vi "HostHoppingScan_v2_MultiRegion.vi"() -> ()   [LabVIEW 2024]
uses:
  <vilib>/Analysis/6fits.llb/Curve Fitting Criteria.ctl
  <vilib>/FPGAPlugInAG/USB-7845R OEM/niLvFpga_Open_USB-7845R OEM.vi
  <vilib>/rvi/interface/common/dynamic/niFpgaDynamicAddResources.vi
  <vilib>/Utility/error.llb/Error Cluster From Error Code.vi
  <vilib>/rvi/errors/niLvFpgaAdjustHostInterfaceError.vi
  <vilib>/rvi/interface/common/niFpgaWaitOnOcc.vi
  <vilib>/FPGAPlugInAG/Dynamic/niLvFpga_Close_Dynamic.vi
  <vilib>/rvi/interface/nirviOpenFPGA/nirviOpenFPGA.xnode
  FPGA Bitfiles/hoppingsicmv2_FPGATarget_FPGAHoppingScanM_mavFg5je4kQ.lvbitx
  <vilib>/rvi/interface/nirviMethod/nirviMethod.xnode
  <vilib>/rvi/interface/nirviReadWriteControl/nirviReadWriteControl.xnode
  <vilib>/rvi/interface/nirviCloseFPGA/nirviCloseFPGA.xnode
  NiFpgaLv.dll
  <vilib>/rvi/interface/Simulation/niFpgaSimulationCallBeginRW.vi
  <vilib>/rvi/errors/niLvFpgaMergeErrorWithErrorCode.vi
  <vilib>/FPGAPlugInAG/Dynamic/niLvFpga_ReadFifo_Dynamic.vi
  <vilib>/FPGAPlugInAG/Dynamic/niLvFpga_WriteFifo_Dynamic.vi
  <vilib>/Analysis/NI_AALPro.lvlib
  <vilib>/FPGAPlugInAG/Dynamic/niLvFpga_ConfigureFifo_Dynamic.vi
panel:
  out "RegionScanning":string
  in  "Auto Image \nSegmentation?":bool
  out "Adapted_YOffset um":dbl format="%#_13g"
  out "Adapted_XOffset um":dbl format="%#_13g"
  out "Adapted_YNum":i32
  out "Adapted_XNum":i32
  in  "Scanning Settings":T1(tab)
  in  "Retract (edge) um":dbl format="%#_13g"
  in  "FrameNum":u32
  in  "XNum":i32
  in  "YNum":i32
  in  "FF_Threshold %":dbl format="%#_13g"
  in  "XStepSize um":dbl format="%#_13g"
  in  "YStepSize um":dbl format="%#_13g"
  in  "YOffset um":dbl format="%#_13g"
  in  "XOffset um":dbl format="%#_13g"
  in  "Retract (flat) um":dbl format="%#_13g"
  in  "RetRate um/s":dbl format="%#_13g"
  in  "FF_AppRate um/s":dbl format="%#_13g"
  in  "NF_AppRate um/s":dbl format="%#_13g"
  in  "Pressure kPa":dbl format="%#_13g"
  in  "NF_Threshold %":dbl format="%#_13g"
  in  "CoordCalThreshold %":dbl format="%#_13g"
  in  "CoordCalRetract um":dbl format="%#_13g"
  in  "YCoordCalEnd um":dbl format="%#_13g"
  in  "XCoordCalEnd um":dbl format="%#_13g"
  in  "YCoordCalBegin um":dbl format="%#_13g"
  in  "XCoordCalBegin um":dbl format="%#_13g"
  in  "CoordCalAppRate um/s":dbl format="%#_13g"
  in  "CoordCalRetRate um/s":dbl format="%#_13g"
  in  "ScanMode":i32(knob) min=0 max=3 scale=0.0..3.0
  out "Signal Size":i32
  out "Done?":bool
  out "HTT_Buffer_Write":u32
  out "Scanned Points":i32
  in  "stop":bool
  in  "Notes":string
  in  "GraphTab":T2(tab)
  out "Topography":dbl[][](graph)
  out "Retract Map":dbl[][](graph)
  out "IZCurve":cluster{dbl[], dbl[]}(graph)
  out "Pressure Slope Map":dbl[][](graph)
  out "FPGA_Host_Buf_Depth":u32
  # "Calibrated Scan\n(New Calibration)"
  # "Calibrated Scan\n(Last Calibration)"
  # "Normal Scan"
  # "Background\nSubstrate Scan"
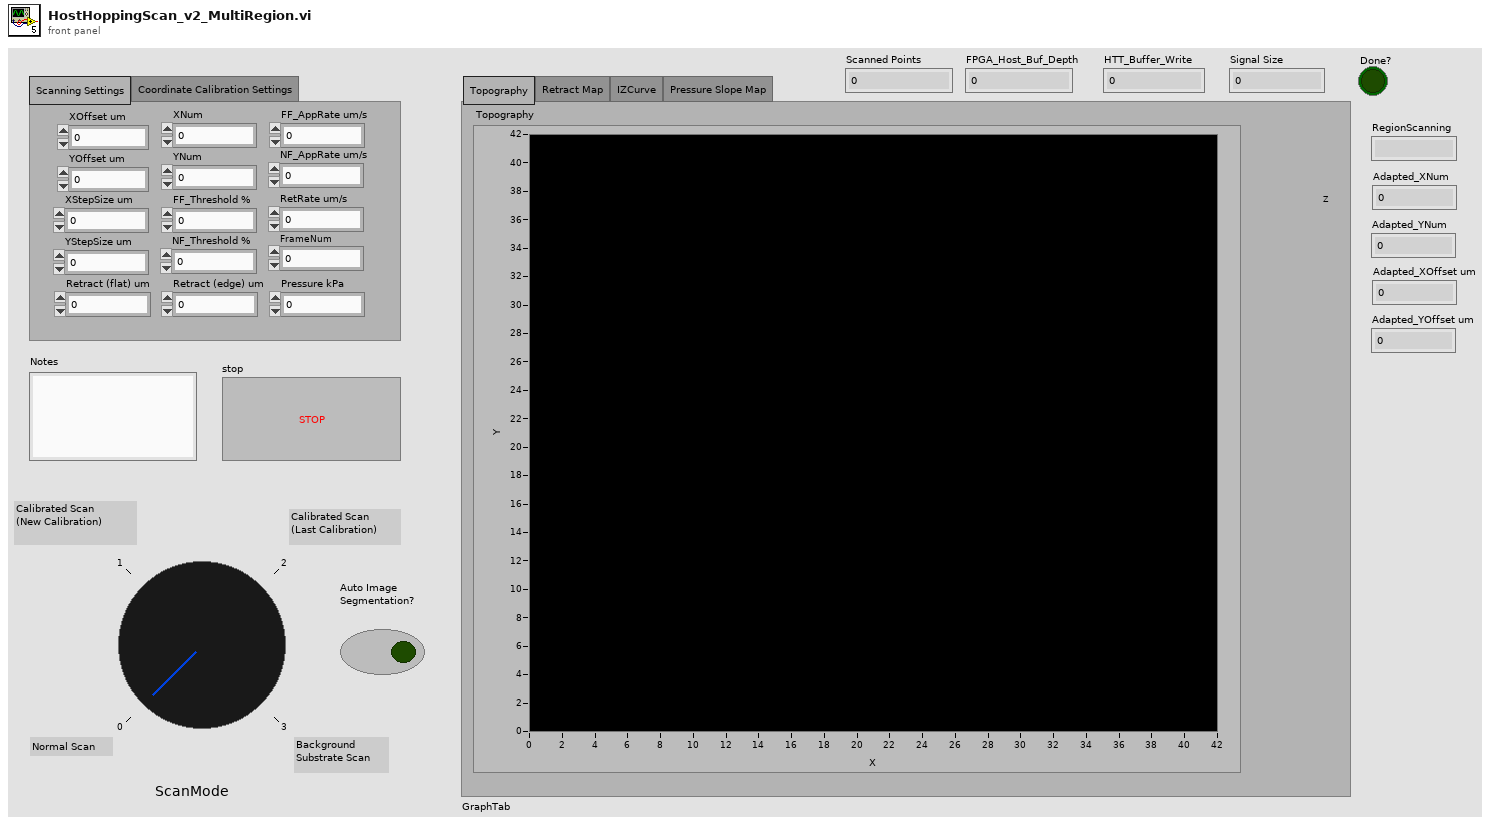
[diagram p1: front panel]
types:
  T1 = enum32{"Scanning Settings", "Coordinate Calibration Settings"}
  T2 = enum32{"Topography", "Retract Map", "IZCurve", "Pressure Slope Map"}
  T3 = typedef "NI_AALPro.lvlib/Curve Fitting Criteria.ctl" = u16
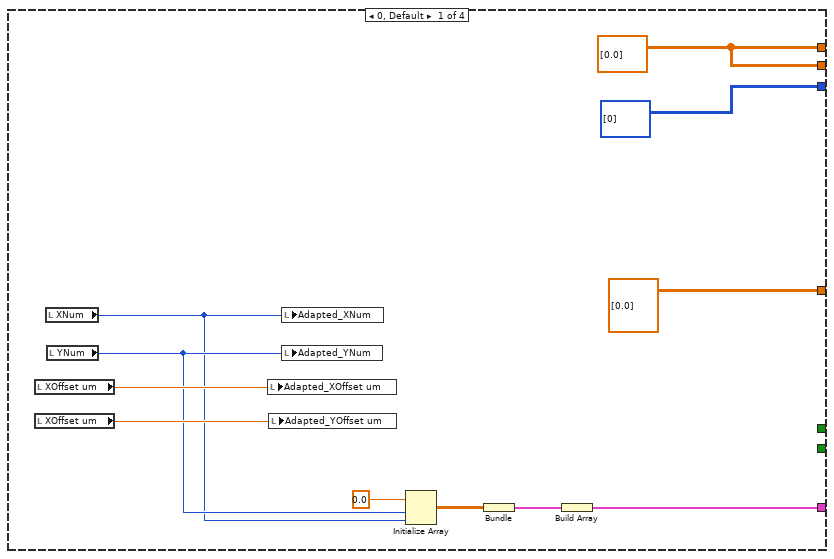
[diagram p3: hidden frame]
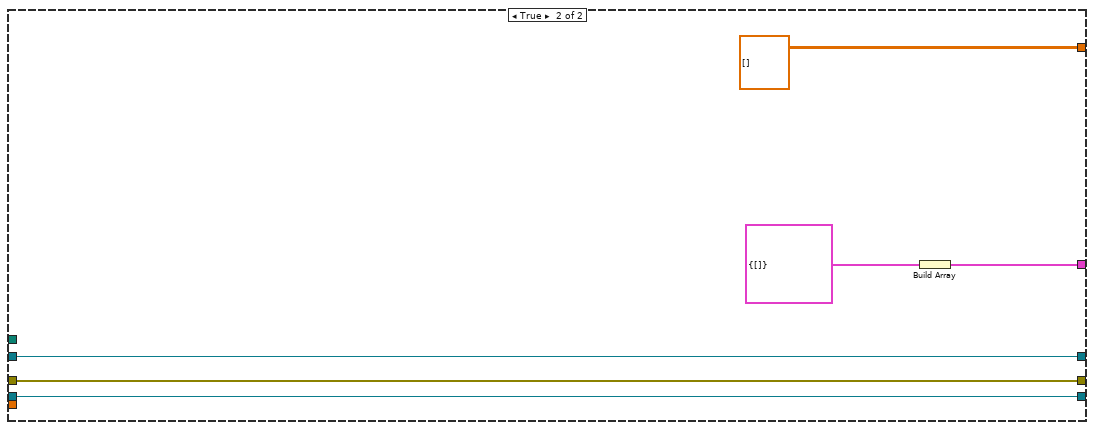
[diagram p4: hidden frame]
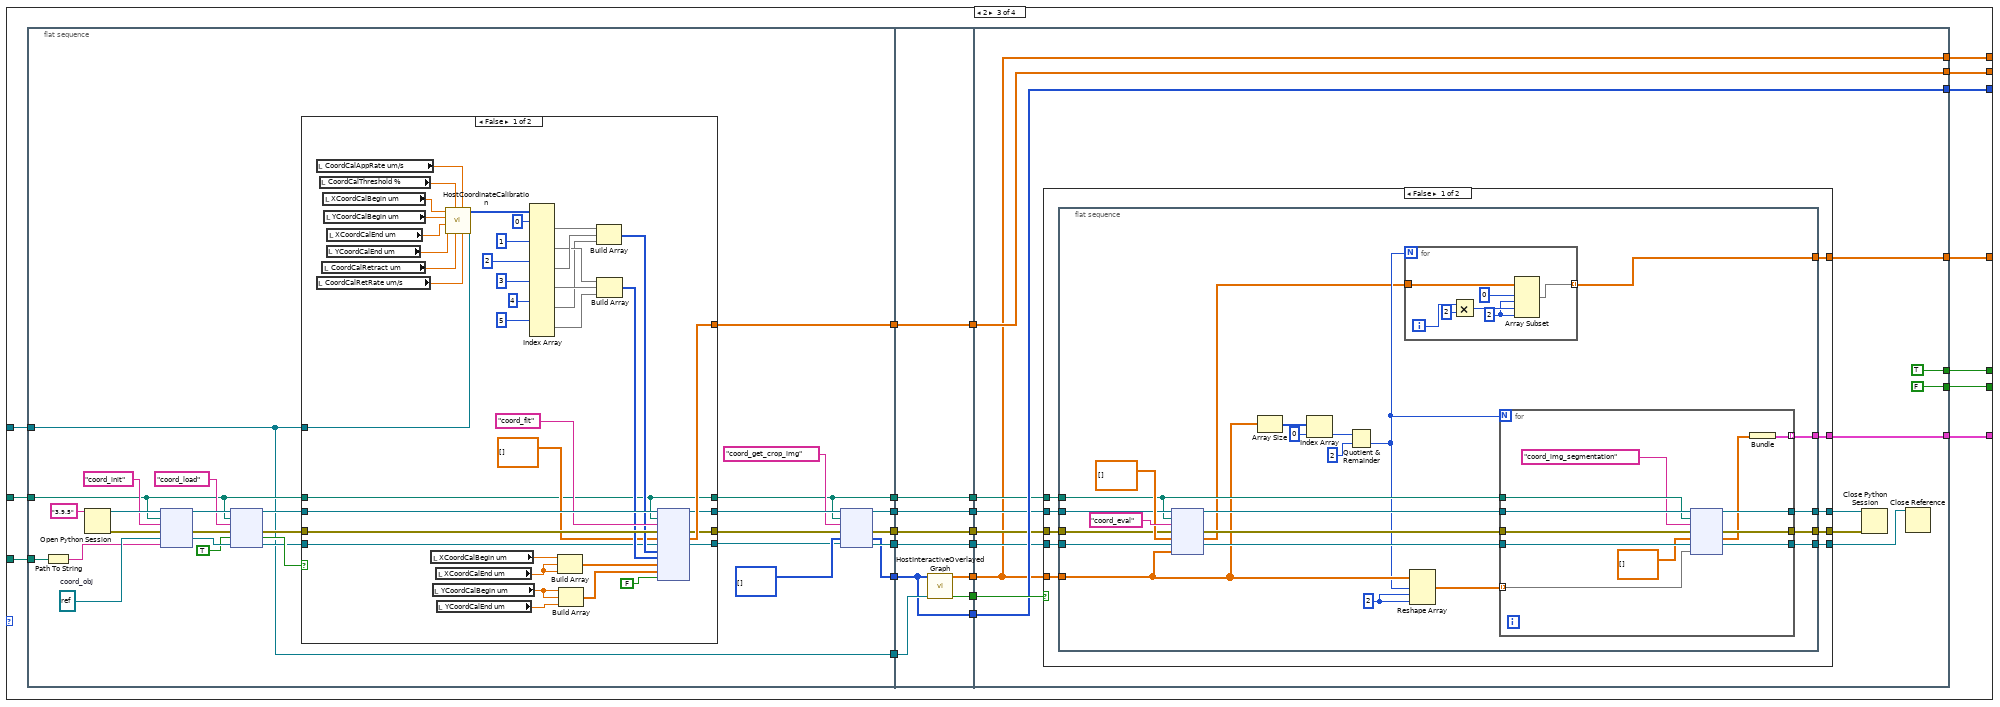
[diagram p5: hidden frame]
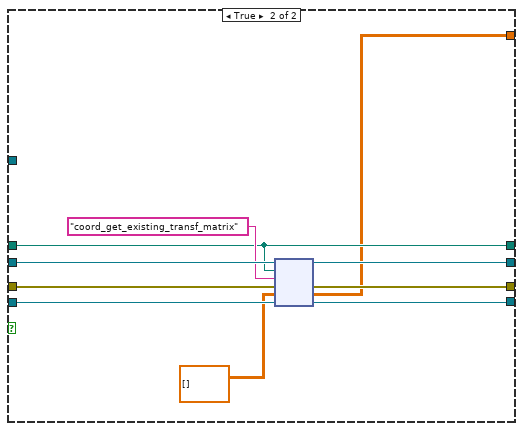
[diagram p6: hidden frame]
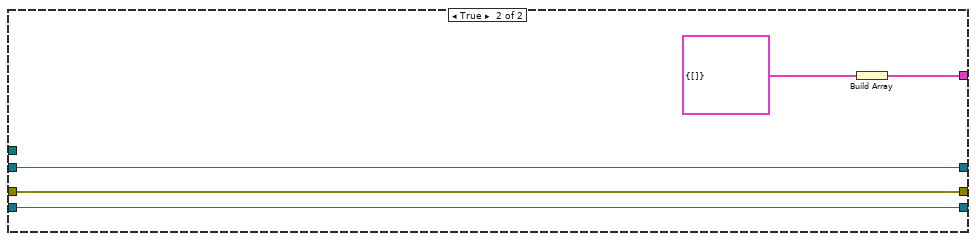
[diagram p7: hidden frame]
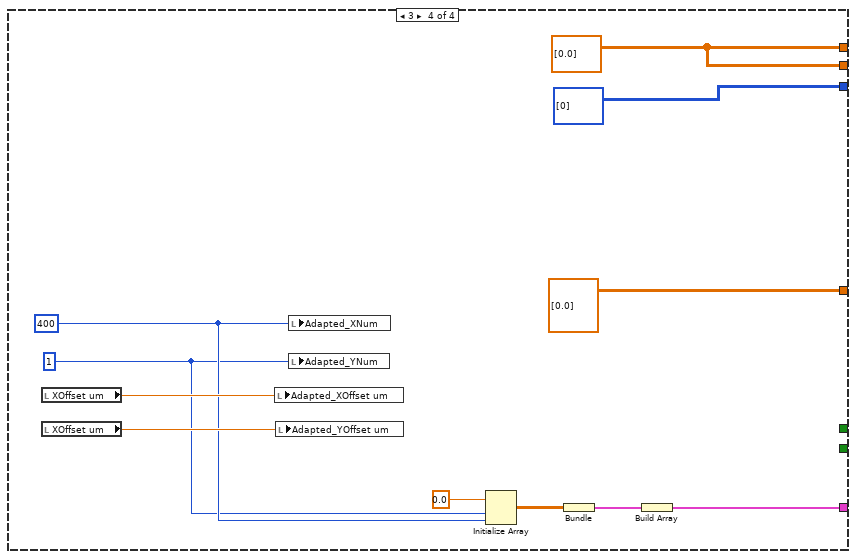
[diagram p8: hidden frame]
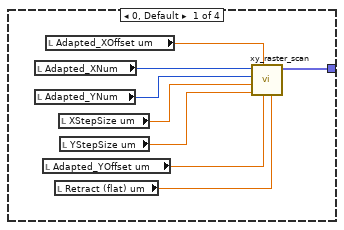
[diagram p14: hidden frame]
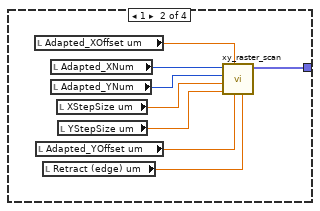
[diagram p15: hidden frame]
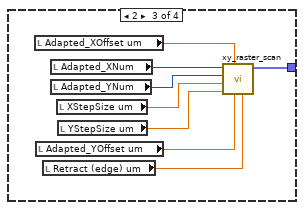
[diagram p16: hidden frame]
diagram:
  n1 = flat-sequence {
    tunnel: [w4] -> w2
    tunnel: w2 -> [w30]
    tunnel: [w27] -> w1
    tunnel: w1 -> [w1436]
    frame #0 {
      n2 = Obtain Queue(max queue size (-1, unlimited)=64, name (unnamed)="stop_sign", element data type=FALSE) -> (queue out=w4:refnum<queue>)  [unwired: 2 in, 2 out]
    }
    frame #1 {
      n3 = flat-sequence {
        tunnel: [w52] -> w31
        tunnel: w30 -> [w52]
        tunnel: w31 -> [w58]
        tunnel: [w58] -> w25
        tunnel: [w54] -> w24
        tunnel: [w107] -> w22
        tunnel: [w108] -> w21
        tunnel: [w109] -> w20
        tunnel: [w110] -> w19
        tunnel: [w111] -> w18
        tunnel: [w74] -> w17
        tunnel: w24 -> [w92]
        tunnel: w25 -> [w74]
        tunnel: [w72] -> w16
        tunnel: [w499] -> w39
        tunnel: [w497] -> w38
        tunnel: [w496] -> w37
        tunnel: [w498] -> w36
        tunnel: [w501] -> w29
        tunnel: w22 -> [w496]
        tunnel: w21 -> [w497]
        tunnel: w20 -> [w499]
        tunnel: w19 -> [w498]
        tunnel: w18 -> [w490]
        tunnel: [w490] -> w23
        tunnel: w17 -> [w494]
        tunnel: w16 -> [w491]
        tunnel: [w491] -> w15
        tunnel: [w489] -> w14
        tunnel: w39 -> [w526]
        tunnel: w38 -> [w525]
        tunnel: w37 -> [w524]
        tunnel: [w522] -> w35
        tunnel: [w521] -> w34
        tunnel: [w520] -> w33
        tunnel: [w519] -> w32
        tunnel: w36 -> [w523]
        tunnel: w29 -> [w518]
        tunnel: [w517] -> w28
        tunnel: w23 -> [w516]
        tunnel: w15 -> [w515]
        tunnel: w14 -> [w514]
        tunnel: [w514] -> w13
        tunnel: [w513] -> w12
        tunnel: [w512] -> w11
        tunnel: [w511] -> w10
        tunnel: [w510] -> w9
        tunnel: [w509] -> w8
        tunnel: [w508] -> w7
        tunnel: w35 -> [w1422]
        tunnel: w34 -> [w1428]
        tunnel: w33 -> [w1427]
        tunnel: w32 -> [w1426]
        tunnel: w28 -> [w1420]
        tunnel: [w1420] -> w26
        tunnel: w13 -> [w1410]
        tunnel: w12 -> [w1409]
        tunnel: w11 -> [w1408]
        tunnel: w10 -> [w1407]
        tunnel: w9 -> [w1406]
        tunnel: w8 -> [w1405]
        tunnel: w7 -> [w1404]
        tunnel: [w1435] -> w27
        tunnel: w26 -> [w1435]
        frame #0 {
          n4 = Wait (ms)(milliseconds to wait=u32 100) -> ()  [unwired: 1 out]
          "Done?" <- FALSE ("Done?")
          "Adapted_XNum" <- "XNum"
          "Adapted_YNum" <- "YNum"
          "Adapted_XOffset um" <- "XStepSize um"
          "Adapted_YOffset um" <- "YStepSize um"
        }
        frame #1 {
          n5 = call "File Dialog"("prompt"="Choose a path to save scanning image data files") -> ("selected path"=w54:path, "cancelled"=w56:bool, "error out"=w55:errorcluster)  [unwired: 11 in, 1 out]
          n6 = Stop(stop? (T)=w56) -> ()
          n7 = call <vilib>:"Clear Errors.vi"("error in (no error)"=w55) -> ()  [unwired: 5 in, 2 out]
        }
        frame #2 {
          w73 = refnum<k38> refnum  # db_obj
          # "coordinate calibration"
          # "use python to save data this time"
          n8 = Path To String(path=w92) -> (string=w106:string)
          n9 = local read "ScanMode"() -> (w75:i32)
          n10 = Get Queue Status(queue=w74) -> (# elements in queue=w91:i32)  [unwired: 2 in, 7 out]
          n11 = Concatenate Strings(w106, "_data.db" ("string")) -> (w105:string)
          n12 = Current VI's Path() -> (path=w97:path)
          n13 = Less Or Equal To 0?(x=w91) -> (x <= 0?=w90:bool)
          n14 = String To Path(string=w105) -> (path=w103:path)
          n15 = Strip Path(path=w97) -> (stripped path=w85:path)  [unwired: 1 out]
          n16 = call <vilib>:"Check if File or Folder Exists.vi"("path"=w103) -> ("file or folder exists?"=w104:bool)  [unwired: 8 in, 2 out]
          n17 = Build Path(base path=w85, name or relative path=path "py/coord_transform.py") -> (appended path=w87:path)
          n18 = Build Path(base path=w85, name or relative path=path "coordinate_calibration/tmp_calibrated_coord") -> (appended path=w84:path)
          n19 = Select(t=w75, s=w90, f=0 ("t")) -> (s? t:f=w89:i32)
          n20 = Build Path(base path=w85, name or relative path=path "py/data_db_arrangement_multi_region.py") -> (appended path=w110:path)
          n21 = case shown="1" w89 {
            tunnel: w87 -> [_ w145 w313 _]
            tunnel: w84 -> [_ w147 w312 _]
            tunnel: w74 -> [_ w146 w311 _]
            tunnel: [w120 w144 w290 w477] -> w111
            tunnel: [i32[][] [[0]] w143 w292 i32[][] [[0]]] -> w60
            tunnel: [w119 w142 w291 w485] -> w61
            tunnel: [w119 w141 w293 w485] -> w62
            tunnel: [_ w140 w294 _] -> w63
            tunnel: [_ w139 w295 _] -> w64
            tunnel: [dbl[][][] [[[0.0]]] ("OutputRetractMap um") w123 w289 dbl[][][] [[[0.0]]] ("OutputRetractMap um")] -> w72
            frame 0, Default {
              w119 = dbl[][] [[0.0]] ("Output_Coord")
              n22 = local read "XOffset um"() -> (w122:dbl)
              n23 = local read "XOffset um"() -> (w121:dbl)
              n24 = local read "XNum"() -> (w112:i32)
              n25 = local read "YNum"() -> (w113:i32)
              n26 = local write "Adapted_XOffset um"(w122) -> ()
              n27 = local write "Adapted_YOffset um"(w121) -> ()
              n28 = local write "Adapted_XNum"(w112) -> ()
              n29 = local write "Adapted_YNum"(w113) -> ()
              n30 = Initialize Array(0.0, w113, w112) -> (w115:dbl[][])
              n31 = Bundle(w115) -> (w114:cluster{dbl[][]})  [unwired: 1 in]
              n32 = Build Array(w114) -> (w120:cluster{dbl[][]}[])
            }
            frame 1 {
              n33 = flat-sequence {
                tunnel: w147 -> [w196]
                tunnel: w146 -> [w149]
                tunnel: w145 -> [w152]
                tunnel: [w152] -> w129
                tunnel: [w160] -> w131
                tunnel: [w155] -> w133
                tunnel: [w154] -> w135
                tunnel: [w153] -> w136
                tunnel: [w150] -> w138
                tunnel: [w149] -> w127
                tunnel: w138 -> [w210]
                tunnel: [w210] -> w137
                tunnel: w136 -> [w202]
                tunnel: w135 -> [w209]
                tunnel: [w209] -> w134
                tunnel: w133 -> [w208]
                tunnel: [w208] -> w132
                tunnel: w131 -> [w207]
                tunnel: [w207] -> w130
                tunnel: w129 -> [w206]
                tunnel: [w206] -> w128
                tunnel: w127 -> [w205]
                tunnel: [w204] -> w126
                tunnel: [w203] -> w125
                tunnel: [w202] -> w124
                tunnel: [w222] -> w144
                tunnel: [w212] -> w143
                tunnel: [w214] -> w142
                tunnel: [w221] -> w141
                tunnel: [TRUE] -> w140
                tunnel: [FALSE] -> w139
                tunnel: w137 -> [w221]
                tunnel: w134 -> [w216]
                tunnel: w132 -> [w217]
                tunnel: w130 -> [w218]
                tunnel: w128 -> [w215]
                tunnel: w126 -> [w214]
                tunnel: w125 -> [w213]
                tunnel: w124 -> [w212]
                tunnel: [w211] -> w123
                frame #0 {
                  w197 = refnum<k38> refnum  # coord_obj
                  # "extended img bundle"
                  # "retracted img bundle"
                  n34 = Path To String(path=w196) -> (string=w195:string)
                  n35 = local read "CoordCalAppRate um/s"() -> (w189:dbl)
                  n36 = local read "CoordCalRetRate um/s"() -> (w187:dbl)
                  n37 = local read "CoordCalThreshold %"() -> (w190:dbl)
                  n38 = local read "CoordCalRetract um"() -> (w188:dbl)
                  n39 = local read "XCoordCalBegin um"() -> (w194:dbl)
                  n40 = local read "YCoordCalBegin um"() -> (w193:dbl)
                  n41 = local read "YCoordCalEnd um"() -> (w191:dbl)
                  n42 = local read "XCoordCalEnd um"() -> (w192:dbl)
                  n43 = Open Python Session(python version="3.9.5" ("Python version")) -> (session out=w200:refnum<k35>, error out=w199:errorcluster)  [unwired: 2 in]
                  n44 = node(w200, w152, "coord_init" ("Python version"), w199, w197, w195) -> (w174:refnum<k35>, w172:errorcluster, w173:refnum<k38>)  [unwired: 1 in, 2 out]
                  n45 = call "HostCoordinateCalibration.vi"("stop_sign_queue"=w149, "RetRate um/s"=w187, "AppRate um/s"=w189, "Retract um"=w188, "Threshold %"=w190, "YCalibrationEnd um"=w191, "XCalibrationEnd um"=w192, "YCalibrationOffset um"=w193, "XCalibrationOffset um"=w194) -> ("img_bundle"=w186:i32[][][])  [unwired: 2 in]
                  n46 = local read "XCoordCalBegin um"() -> (w169:dbl)
                  n47 = local read "YCoordCalBegin um"() -> (w166:dbl)
                  n48 = local read "XCoordCalEnd um"() -> (w168:dbl)
                  n49 = local read "YCoordCalEnd um"() -> (w167:dbl)
                  n50 = Index Array(array=w186, index (dim 0) #1=0 ("index (page)"), index (dim 0) #2=1 ("index (page)"), index (dim 0) #3=2 ("index (page)"), index (dim 0) #4=3 ("index (page)"), index (dim 0) #5=4 ("index (page)"), index (dim 0) #6=5 ("index (page)")) -> (element #1=w148:i32[][], element #2=w178:i32[][], element #3=w179:i32[][], element #4=w177:i32[][], element #5=w176:i32[][], element #6=w175:i32[][])  [unwired: 12 in]
                  n51 = Build Array(w169, w168, w168) -> (w165:dbl[])
                  n52 = Build Array(w166, w166, w167) -> (w164:dbl[])
                  n53 = Build Array(w148, w179, w176) -> (w171:i32[][][])
                  n54 = Build Array(w178, w177, w175) -> (w170:i32[][][])
                  n55 = node(w174, w152, "coord_fit" ("function name"), w172, dbl[][] [], w173, w171, w170, w165, w164, TRUE) -> (w161:refnum<k35>, w159:errorcluster, w150:dbl[][], w157:refnum<k38>)  [unwired: 5 in, 2 out]
                  n56 = node(w161, w152, "coord_get_crop_img" ("function name"), w159, i32[][] [], w157) -> (w160:refnum<k35>, w155:errorcluster, w153:i32[][], w154:refnum<k38>)  [unwired: 2 out]
                }
                frame #1 {
                  n57 = call "HostInteractiveOverlayedGraph.vi"("stop_sign_queue"=w205, "InputImg"=w202) -> ("Break"=w203:bool, "Output_Coord"=w204:dbl[][])  [unwired: 8 in]
                }
                frame #2 {
                  n58 = case shown="False" w213 {
                    tunnel: [w235 w288] -> w225
                    tunnel: [w234 w287] -> w224
                    tunnel: [w233 w286] -> w223
                    tunnel: [w227 w283] -> w222
                    tunnel: w214 -> [w232 _]
                    tunnel: w218 -> [w231 w288]
                    tunnel: w217 -> [w230 w287]
                    tunnel: w216 -> [w229 w286]
                    tunnel: w215 -> [w228 _]
                    tunnel: [w226 dbl[][][] [] ("OutputRetractMap um")] -> w211
                    frame False {
                      n59 = flat-sequence {
                        tunnel: [w245] -> w227
                        tunnel: [w255] -> w233
                        tunnel: [w256] -> w234
                        tunnel: [w257] -> w235
                        tunnel: w228 -> [w246]
                        tunnel: w229 -> [w252]
                        tunnel: w230 -> [w253]
                        tunnel: w231 -> [w254]
                        tunnel: w232 -> [w237]
                        tunnel: [w239] -> w226
                        frame #0 {
                          n60 = node(w254, w246, "coord_eval" ("function name"), w253, dbl[][] [], w252, w237) -> (w249:refnum<k35>, w248:errorcluster, w240:dbl[][], w247:refnum<k38>)  [unwired: 1 in, 2 out]
                          n61 = Array Size(array=w237) -> (size(s)=w244:i32[])
                          n62 = Index Array(array=w244, index=0) -> (element=w242:i32)
                          n63 = Quotient & Remainder(x=w242, y=2 ("index")) -> (floor(x/y)=w238:i32)  [unwired: 1 out]
                          n64 = for {
                            N: w238 -> [_]
                            tunnel: w237 -> [w263]
                            tunnel: [w258] -> w236 mode=indexing
                            i -> [w262]
                            n65 = Multiply(x=w262, y=2) -> (x*y=w260:i32)
                            n66 = Array Subset(array=w263, index (row)=w260, length (row)=2 ("length")) -> (w258:dbl[][])  [unwired: 2 in]
                          }
                          n67 = for {
                            N: w238 -> [_]
                            tunnel: w240 -> [w267]
                            tunnel: [w266] -> w239 mode=indexing
                            i -> [w264]
                            w268 = 2 ("length")
                            n68 = Multiply(x=2 ("y"), y=w264) -> (x*y=w270:i32)
                            n69 = Array Subset(array=w267, index (row)=0 ("index"), length (row)=w268, index (col)=w270, length (col)=w268) -> (w266:dbl[][])
                          }
                          n70 = for {
                            N: w238 -> [_]
                            tunnel: w236 -> [w279] mode=indexing
                            tunnel: w246 -> [w273]
                            tunnel: [w271] -> w245 mode=indexing
                            tunnel: w249 -> [w278]
                            tunnel: [w282] -> w257
                            tunnel: w248 -> [w277]
                            tunnel: [w281] -> w256
                            tunnel: w247 -> [w276]
                            tunnel: [w280] -> w255
                            n71 = node(w278, w273, "coord_img_segmentation" ("function name"), w277, dbl[][] [], w276, w279) -> (w282:refnum<k35>, w281:errorcluster, w272:dbl[][], w280:refnum<k38>)  [unwired: 1 in, 2 out]
                            n72 = Bundle(w272) -> (w271:cluster{dbl[][]})  [unwired: 1 in]
                          }
                        }
                      }
                    }
                    frame True {
                      n73 = Build Array(cluster{dbl[][]} {[]}) -> (w283:cluster{dbl[][]}[])
                    }
                  }
                  n74 = Close Python Session(session in=w225, error in=w224) -> ()  [unwired: 1 out]
                  n75 = Close Reference(reference=w223) -> ()  [unwired: 1 in, 1 out]
                }
              }
            }
            frame 2 {
              n76 = flat-sequence {
                tunnel: w313 -> [w327]
                tunnel: w312 -> [w336]
                tunnel: w311 -> [w325]
                tunnel: [w314] -> w310
                tunnel: [w325] -> w309
                tunnel: [w324] -> w308
                tunnel: [w318] -> w305
                tunnel: [w317] -> w303
                tunnel: [w316] -> w301
                tunnel: [w315] -> w299
                tunnel: w310 -> [w394]
                tunnel: w309 -> [w402]
                tunnel: w308 -> [w401]
                tunnel: [w401] -> w307
                tunnel: [w400] -> w306
                tunnel: w305 -> [w400]
                tunnel: [w399] -> w304
                tunnel: w303 -> [w399]
                tunnel: [w398] -> w302
                tunnel: w301 -> [w398]
                tunnel: [w397] -> w300
                tunnel: w299 -> [w397]
                tunnel: [w396] -> w298
                tunnel: [w395] -> w297
                tunnel: [w394] -> w296
                tunnel: w307 -> [w414]
                tunnel: w306 -> [w412]
                tunnel: w304 -> [w411]
                tunnel: w302 -> [w410]
                tunnel: w300 -> [w409]
                tunnel: w298 -> [w408]
                tunnel: w297 -> [w417]
                tunnel: w296 -> [w413]
                tunnel: [FALSE] -> w295
                tunnel: [TRUE] -> w294
                tunnel: [w414] -> w293
                tunnel: [w413] -> w292
                tunnel: [w408] -> w291
                tunnel: [w404] -> w290
                tunnel: [w403] -> w289
                frame #0 {
                  w338 = refnum<k38> refnum  # coord_obj
                  n77 = Path To String(path=w336) -> (string=w337:string)
                  n78 = Open Python Session(python version="3.9.5" ("Python version")) -> (session out=w341:refnum<k35>, error out=w340:errorcluster)  [unwired: 2 in]
                  n79 = node(w341, w327, "coord_init" ("Python version"), w340, w338, w337) -> (w335:refnum<k35>, w334:errorcluster, w333:refnum<k38>)  [unwired: 1 in, 2 out]
                  n80 = node(w335, w327, "coord_load" ("Python version"), w334, TRUE, w333) -> (w329:refnum<k35>, w328:errorcluster, w330:bool, w326:refnum<k38>)  [unwired: 2 out]
                  n81 = case shown="False" w330 {
                    tunnel: w329 -> [w361 w393]
                    tunnel: w328 -> [w359 w392]
                    tunnel: w325 -> [w375 _]
                    tunnel: w327 -> [w343 w385]
                    tunnel: w326 -> [w349 w391]
                    tunnel: [w347 w384] -> w324
                    tunnel: [w346 w388] -> w323
                    tunnel: [w345 w387] -> w320
                    tunnel: [w344 w386] -> w319
                    tunnel: [w343 w385] -> w318
                    frame False {
                      n82 = local read "CoordCalAppRate um/s"() -> (w378:dbl)
                      n83 = local read "CoordCalRetRate um/s"() -> (w376:dbl)
                      n84 = local read "CoordCalThreshold %"() -> (w379:dbl)
                      n85 = local read "CoordCalRetract um"() -> (w377:dbl)
                      n86 = local read "XCoordCalBegin um"() -> (w383:dbl)
                      n87 = local read "YCoordCalBegin um"() -> (w382:dbl)
                      n88 = local read "YCoordCalEnd um"() -> (w380:dbl)
                      n89 = local read "XCoordCalEnd um"() -> (w381:dbl)
                      n90 = local read "XCoordCalBegin um"() -> (w358:dbl)
                      n91 = local read "YCoordCalBegin um"() -> (w355:dbl)
                      n92 = local read "XCoordCalEnd um"() -> (w357:dbl)
                      n93 = local read "YCoordCalEnd um"() -> (w356:dbl)
                      n94 = call "HostCoordinateCalibration.vi"("stop_sign_queue"=w375, "RetRate um/s"=w376, "AppRate um/s"=w378, "Retract um"=w377, "Threshold %"=w379, "YCalibrationEnd um"=w380, "XCalibrationEnd um"=w381, "YCalibrationOffset um"=w382, "XCalibrationOffset um"=w383) -> ("img_bundle"=w362:i32[][][])  [unwired: 2 in]
                      n95 = Index Array(array=w362, index (dim 0) #1=0 ("index (page)"), index (dim 0) #2=1 ("index (page)"), index (dim 0) #3=2 ("index (page)"), index (dim 0) #4=3 ("index (page)"), index (dim 0) #5=4 ("index (page)"), index (dim 0) #6=5 ("index (page)")) -> (element #1=w363:i32[][], element #2=w367:i32[][], element #3=w368:i32[][], element #4=w366:i32[][], element #5=w365:i32[][], element #6=w364:i32[][])  [unwired: 12 in]
                      n96 = Build Array(w358, w357, w357) -> (w352:dbl[])
                      n97 = Build Array(w355, w355, w356) -> (w351:dbl[])
                      n98 = Build Array(w363, w368, w365) -> (w354:i32[][][])
                      n99 = Build Array(w367, w366, w364) -> (w353:i32[][][])
                      n100 = node(w361, w343, "coord_fit" ("function name"), w359, dbl[][] [], w349, w354, w353, w352, w351, FALSE) -> (w346:refnum<k35>, w345:errorcluster, w347:dbl[][], w344:refnum<k38>)  [unwired: 5 in, 2 out]
                    }
                    frame True {
                      n101 = node(w393, w385, "coord_get_existing_transf_matrix" ("Python version"), w392, dbl[][] [], w391) -> (w388:refnum<k35>, w387:errorcluster, w384:dbl[][], w386:refnum<k38>)  [unwired: 2 out]
                    }
                  }
                  n102 = node(w323, w318, "coord_get_crop_img" ("function name"), w320, i32[][] [], w319) -> (w317:refnum<k35>, w316:errorcluster, w314:i32[][], w315:refnum<k38>)  [unwired: 2 out]
                }
                frame #1 {
                  n103 = call "HostInteractiveOverlayedGraph.vi"("stop_sign_queue"=w402, "InputImg"=w394) -> ("Break"=w395:bool, "Output_Coord"=w396:dbl[][])  [unwired: 8 in]
                }
                frame #2 {
                  n104 = case shown="False" w417 {
                    tunnel: w412 -> [w427 _]
                    tunnel: w411 -> [w426 w474]
                    tunnel: w410 -> [w425 w473]
                    tunnel: w409 -> [w424 w472]
                    tunnel: w408 -> [w423 _]
                    tunnel: [w422 w474] -> w407
                    tunnel: [w421 w473] -> w406
                    tunnel: [w420 w472] -> w405
                    tunnel: [w419 w470] -> w404
                    tunnel: [w418 _] -> w403
                    frame False {
                      n105 = flat-sequence {
                        tunnel: [w450] -> w422
                        tunnel: [w449] -> w421
                        tunnel: [w448] -> w420
                        tunnel: [w447] -> w419
                        tunnel: w423 -> [w432]
                        tunnel: w424 -> [w442]
                        tunnel: w425 -> [w443]
                        tunnel: w426 -> [w444]
                        tunnel: w427 -> [w438]
                        tunnel: [w429] -> w418
                        frame #0 {
                          w433 = 2 ("index")
                          n106 = node(w444, w438, "coord_eval" ("function name"), w443, dbl[][] [], w442, w432) -> (w441:refnum<k35>, w440:errorcluster, w428:dbl[][], w439:refnum<k38>)  [unwired: 1 in, 2 out]
                          n107 = Array Size(array=w432) -> (size(s)=w437:i32[])
                          n108 = Index Array(array=w437, index=0) -> (element=w435:i32)
                          n109 = Quotient & Remainder(x=w435, y=2 ("index")) -> (floor(x/y)=w430:i32)  [unwired: 1 out]
                          n110 = for {
                            N: w430 -> [_]
                            tunnel: w428 -> [w457]
                            tunnel: [w454] -> w429 mode=indexing
                            i -> [w456]
                            w451 = 2 ("length")
                            n111 = Multiply(x=w456, y=2) -> (x*y=w453:i32)
                            n112 = Array Subset(array=w457, index (row)=0 ("index"), length (row)=w451, index (col)=w453, length (col)=w451) -> (w454:dbl[][])
                          }
                          n113 = Reshape Array(w432, w430, w433, w433) -> (w431:dbl[][][])
                          n114 = for {
                            N: w430 -> [_]
                            tunnel: w431 -> [w466] mode=indexing
                            tunnel: w438 -> [w465]
                            tunnel: [w458] -> w447 mode=indexing
                            tunnel: w441 -> [w469]
                            tunnel: [w464] -> w450
                            tunnel: w440 -> [w468]
                            tunnel: [w462] -> w449
                            tunnel: w439 -> [w467]
                            tunnel: [w461] -> w448
                            n115 = node(w469, w465, "coord_img_segmentation" ("function name"), w468, dbl[][] [], w467, w466) -> (w464:refnum<k35>, w462:errorcluster, w459:dbl[][], w461:refnum<k38>)  [unwired: 1 in, 2 out]
                            n116 = Bundle(w459) -> (w458:cluster{dbl[][]})  [unwired: 1 in]
                          }
                        }
                      }
                    }
                    frame True {
                      n117 = Build Array(cluster{dbl[][]} {[]}) -> (w470:cluster{dbl[][]}[])
                    }
                  }
                  n118 = Close Python Session(session in=w407, error in=w406) -> ()  [unwired: 1 out]
                  n119 = Close Reference(reference=w405) -> ()  [unwired: 1 in, 1 out]
                }
              }
            }
            frame 3 {
              w475 = 1 ("Adapted_XNum")
              w476 = 400 ("Adapted_XNum")
              w485 = dbl[][] [[0.0]] ("Output_Coord")
              n120 = local read "XOffset um"() -> (w482:dbl)
              n121 = local read "XOffset um"() -> (w481:dbl)
              n122 = local write "Adapted_XOffset um"(w482) -> ()
              n123 = local write "Adapted_YOffset um"(w481) -> ()
              n124 = local write "Adapted_XNum"(w476) -> ()
              n125 = local write "Adapted_YNum"(w475) -> ()
              n126 = Initialize Array(0.0, w475, w476) -> (w479:dbl[][])
              n127 = Bundle(w479) -> (w478:cluster{dbl[][]})  [unwired: 1 in]
              n128 = Build Array(w478) -> (w477:cluster{dbl[][]}[])
            }
          }
          n129 = case shown="True" w104 {
            tunnel: w103 -> [w486 w488]
            tunnel: [w486 w487] -> w102
            frame False {
            }
            frame True {
              n130 = Delete(path (use dialog)=w488) -> (deleted path=w487:path)  [unwired: 4 in, 2 out]
            }
          }
          n131 = Path To String(path=w102) -> (string=w94:string)
          n132 = Open Python Session(python version="3.9.5" ("Python version")) -> (session out=w99:refnum<k35>, error out=w98:errorcluster)  [unwired: 2 in]
          n133 = node(w99, w110, "db_init" ("Python version"), w98, w73, w94) -> (w83:refnum<k35>, w82:errorcluster, w81:refnum<k38>)  [unwired: 1 in, 2 out]
          n134 = local read "CoordCalAppRate um/s"() -> (w65:dbl)
          n135 = local read "CoordCalRetRate um/s"() -> (w59:dbl)
          n136 = local read "CoordCalThreshold %"() -> (w67:dbl)
          n137 = local read "CoordCalRetract um"() -> (w66:dbl)
          n138 = local read "XCoordCalBegin um"() -> (w71:dbl)
          n139 = local read "YCoordCalBegin um"() -> (w70:dbl)
          n140 = local read "YCoordCalEnd um"() -> (w68:dbl)
          n141 = local read "XCoordCalEnd um"() -> (w69:dbl)
          n142 = node(w83, w110, "db_insert_coordinate_calibration" ("function name"), w82, w81, w71, w70, w69, w68, w67, w66, w65, w59, w60, w61, w62, w63, w64) -> (w80:refnum<k35>, w79:errorcluster, w78:refnum<k38>)  [unwired: 15 in, 2 out]
          n143 = node(w80, w110, "db_start_global_timer" ("function name"), w79, w78) -> (w109:refnum<k35>, w108:errorcluster, w107:refnum<k38>)  [unwired: 2 in, 2 out]
        }
        frame #3 {
          n144 = Get Queue Status(queue=w494) -> (queue out=w493:refnum<queue>, # elements in queue=w495:i32)  [unwired: 2 in, 6 out]
          n145 = Greater Than 0?(x=w495) -> (x > 0?=w492:bool)
          n146 = case shown="True" w492 {
            tunnel: w493 -> [w502 w505]
            tunnel: [w502 w503] -> w501
            frame False {
            }
            frame True {
              n147 = flat-sequence {
                tunnel: w505 -> [w506]
                tunnel: [w506] -> w504
                tunnel: w504 -> [w507]
                tunnel: [w507] -> w503
                frame #0 {
                  n148 = Release Queue(queue=w506) -> ()  [unwired: 2 in, 3 out]
                }
                frame #1 {
                  n149 = Stop() -> ()  [unwired: 1 in]
                }
              }
            }
          }
          n150 = Array Size(array=w490) -> (size(s)=w489:i32)
          n151 = Wait (ms)(milliseconds to wait=u32 200) -> ()  [unwired: 1 out]
        }
        frame #4 {
          n152 = for {
            N: w514 -> [_]
            tunnel: w516 -> [w559] mode=indexing
            tunnel: w523 -> [w566]
            tunnel: [w565] -> w522
            tunnel: w526 -> [w569]
            tunnel: [w564] -> w521
            tunnel: w525 -> [w568]
            tunnel: [w563] -> w520
            tunnel: w524 -> [w567]
            tunnel: [w562] -> w519
            tunnel: w518 -> [w561]
            tunnel: [w560] -> w517
            tunnel: w515 -> [w545] mode=indexing
            tunnel: w514 -> [w541]
            tunnel: [w532] -> w513 mode=indexing
            tunnel: [w531] -> w512 mode=indexing
            tunnel: [w530] -> w511 mode=indexing
            tunnel: [w529] -> w510 mode=indexing
            tunnel: [w528] -> w509 mode=indexing
            tunnel: [w527] -> w508 mode=indexing
            i -> [w544]
            stop <- w546 stop-if-true
            n153 = flat-sequence {
              tunnel: w559 -> [w577]
              tunnel: w561 -> [w586]
              tunnel: w566 -> [w587]
              tunnel: w567 -> [w588]
              tunnel: w568 -> [w589]
              tunnel: w569 -> [w590]
              tunnel: [w590] -> w558
              tunnel: [w589] -> w556
              tunnel: [w588] -> w554
              tunnel: [w587] -> w552
              tunnel: [w586] -> w550
              tunnel: [w576] -> w548
              tunnel: w545 -> [w585]
              tunnel: w544 -> [w582]
              tunnel: [w582] -> w542
              tunnel: w541 -> [w584]
              tunnel: [w584] -> w539
              tunnel: w558 -> [w638]
              tunnel: [w638] -> w557
              tunnel: w556 -> [w637]
              tunnel: [w637] -> w555
              tunnel: w554 -> [w636]
              tunnel: [w636] -> w553
              tunnel: w552 -> [w635]
              tunnel: [w635] -> w551
              tunnel: w550 -> [w634]
              tunnel: [w634] -> w549
              tunnel: w548 -> [w629]
              tunnel: [w628] -> w547
              tunnel: [w627] -> w543
              tunnel: w542 -> [w627]
              tunnel: [w626] -> w540
              tunnel: w539 -> [w626]
              tunnel: w557 -> [w652]
              tunnel: w555 -> [w651]
              tunnel: w553 -> [w650]
              tunnel: w551 -> [w649]
              tunnel: w549 -> [w644]
              tunnel: w547 -> [w642]
              tunnel: w543 -> [w640]
              tunnel: w540 -> [w639]
              tunnel: [w648] -> w538
              tunnel: [w647] -> w537
              tunnel: [w646] -> w536
              tunnel: [w645] -> w535
              tunnel: [w643] -> w534
              tunnel: [w641] -> w533
              tunnel: [w1398] -> w546
              tunnel: [w1399] -> w560
              tunnel: [w1400] -> w562
              tunnel: [w1401] -> w563
              tunnel: [w1402] -> w564
              tunnel: [w1403] -> w565
              tunnel: w538 -> [w1403]
              tunnel: w537 -> [w1402]
              tunnel: w536 -> [w1401]
              tunnel: w535 -> [w1400]
              tunnel: w534 -> [w1399]
              tunnel: w533 -> [w1398]
              tunnel: [w1397] -> w532
              tunnel: [w1396] -> w531
              tunnel: [w1395] -> w530
              tunnel: [w1394] -> w529
              tunnel: [w1393] -> w528
              tunnel: [w1392] -> w527
              frame #0 {
                n154 = local read "ScanMode"() -> (w573:i32)
                n155 = Equal?(x=w573, y=1) -> (x = y?=w572:bool)
                n156 = Equal?(x=w573, y=2) -> (x = y?=w571:bool)
                n157 = Unbundle(w577) -> (w576:dbl[][])
                n158 = Or(x=w572, y=w571) -> (x .or. y?=w570:bool)
                n159 = case shown="True" w570 {
                  tunnel: w585 -> [_ w599]
                  frame False {
                  }
                  frame True {
                    n160 = local read "YCoordCalBegin um"() -> (w617:dbl)
                    n161 = Index Array(array=w599, index (col) #1=0 ("index (row)"), index (col) #2=1 ("index (row)")) -> (element #1=w625:dbl[], element #2=w624:dbl[])  [unwired: 2 in]
                    n162 = local read "YCoordCalEnd um"() -> (w618:dbl)
                    n163 = Index Array(array=w625, index #1=0 ("index"), index #2=1 ("index")) -> (element #1=w623:dbl, element #2=w621:dbl)
                    n164 = Index Array(array=w624, index #1=0 ("index"), index #2=1 ("index")) -> (element #1=w622:dbl, element #2=w620:dbl)
                    n165 = local read "YStepSize um"() -> (w606:dbl)
                    n166 = local read "XStepSize um"() -> (w612:dbl)
                    n167 = Max & Min(x=w623, y=w622) -> (max(x,y)=w614:dbl, min(x,y)=w596:dbl)
                    n168 = Max & Min(x=w621, y=w620) -> (max(x,y)=w597:dbl, min(x,y)=w598:dbl)
                    n169 = Subtract(x=w618, y=w617) -> (x-y=w619:dbl)
                    n170 = Subtract(x=w614, y=w596) -> (x-y=w613:dbl)
                    n171 = Subtract(x=w619, y=w597) -> (x-y=w592:dbl)
                    n172 = Subtract(x=w597, y=w598) -> (x-y=w607:dbl)
                    n173 = Divide(x=w613, y=w612) -> (x/y=w616:dbl)
                    n174 = Divide(x=w607, y=w606) -> (x/y=w608:dbl)
                    n175 = Subtract(x=w596, y=1.0) -> (x-y=w595:dbl)
                    n176 = Subtract(x=w592, y=0.0) -> (x-y=w591:dbl)
                    n177 = Round To Nearest(number=w616) -> (nearest integer value=w615:dbl)
                    n178 = Round To Nearest(number=w608) -> (nearest integer value=w609:dbl)
                    n179 = local write "Adapted_XOffset um"(w595) -> ()
                    n180 = To Long Integer(number=w615) -> (32bit integer=w611:i32)
                    n181 = To Long Integer(number=w609) -> (32bit integer=w610:i32)
                    n182 = local write "Adapted_YOffset um"(w591) -> ()
                    n183 = local write "Adapted_XNum"(w611) -> ()
                    n184 = local write "Adapted_YNum"(w610) -> ()
                  }
                }
                n185 = Increment(x=w582) -> (x+1=w581:i32)
                n186 = Number To Decimal String(number=w584) -> (decimal integer string=w580:string)  [unwired: 1 in]
                n187 = Number To Decimal String(number=w581) -> (decimal integer string=w579:string)  [unwired: 1 in]
                n188 = Concatenate Strings(w579, " / " ("string"), w580) -> (w583:string)
                n189 = local write "RegionScanning"(w583) -> ()
              }
              frame #1 {
                n190 = local read "Adapted_XNum"() -> (w633:i32)
                n191 = local read "Adapted_YNum"() -> (w632:i32)
                n192 = local read "Retract (edge) um"() -> (w630:dbl)
                n193 = local read "Retract (flat) um"() -> (w631:dbl)
                n194 = call "HostDynamicRetractFormalization.vi"("Retract_Edge um"=w630, "Retract_Flat um"=w631, "YNum"=w632, "XNum"=w633, "InputLabel"=w629) -> ("OutputRetractMap um"=w628:dbl[][])  [unwired: 6 in]
                n195 = local write "Retract Map"(w628) -> ()
              }
              frame #2 {
                n196 = local read "FrameNum"() -> (w653:u32)
                n197 = for {
                  N: w653 -> [_]
                  tunnel: w652 -> [w687]
                  tunnel: w651 -> [w686]
                  tunnel: w650 -> [w685]
                  tunnel: w649 -> [w684]
                  tunnel: [w673] -> w648
                  tunnel: [w672] -> w647
                  tunnel: [w671] -> w646
                  tunnel: [w670] -> w645
                  tunnel: w644 -> [w667]
                  tunnel: [w664] -> w643
                  tunnel: w642 -> [w661]
                  tunnel: [w659] -> w641
                  tunnel: w640 -> [w658]
                  tunnel: w639 -> [w656]
                  i -> [w683]
                  stop <- w659 stop-if-true
                  n198 = flat-sequence {
                    tunnel: w683 -> [w706]
                    tunnel: w684 -> [w699]
                    tunnel: w685 -> [w701]
                    tunnel: w686 -> [w702]
                    tunnel: w687 -> [w703]
                    tunnel: [w700] -> w682
                    tunnel: [w698] -> w681
                    tunnel: [w697] -> w680
                    tunnel: [w699] -> w679
                    tunnel: [w706] -> w678
                    tunnel: w667 -> [w695]
                    tunnel: [w695] -> w666
                    tunnel: w661 -> [w693]
                    tunnel: [w693] -> w660
                    tunnel: w658 -> [w690]
                    tunnel: [w690] -> w657
                    tunnel: w656 -> [w689]
                    tunnel: [w689] -> w655
                    tunnel: [w752] -> w688
                    tunnel: w682 -> [w747]
                    tunnel: w681 -> [w746]
                    tunnel: w680 -> [w745]
                    tunnel: w679 -> [w744]
                    tunnel: w678 -> [w712]
                    tunnel: [w739] -> w677
                    tunnel: [w738] -> w676
                    tunnel: [w737] -> w675
                    tunnel: [w736] -> w674
                    tunnel: [w735] -> w669
                    tunnel: [w734] -> w668
                    tunnel: w666 -> [w724]
                    tunnel: [w723] -> w665
                    tunnel: [w719] -> w663
                    tunnel: [w718] -> w662
                    tunnel: w660 -> [w713]
                    tunnel: w657 -> [w711]
                    tunnel: w655 -> [w710]
                    tunnel: [w707] -> w654
                    tunnel: w688 -> [w1391]
                    tunnel: w677 -> [w1386]
                    tunnel: w676 -> [w1388]
                    tunnel: w675 -> [w1387]
                    tunnel: w674 -> [w1383]
                    tunnel: [w1386] -> w673
                    tunnel: [w1385] -> w672
                    tunnel: [w1384] -> w671
                    tunnel: [w1382] -> w670
                    tunnel: w669 -> [w1389]
                    tunnel: w668 -> [w1390]
                    tunnel: [w1390] -> w659
                    tunnel: w665 -> [w1380]
                    tunnel: [w1380] -> w664
                    tunnel: w663 -> [w1379]
                    tunnel: w662 -> [w1378]
                    tunnel: w654 -> [w1377]
                    frame #0 {
                      w691 = u8 2 ("Z Scale.Scale Fit")
                      w692 = TRUE ("Smooth Update")
                      w694 = FALSE ("Y Scale.Loose Fit")
                      n199 = local read "Adapted_YNum"() -> (w704:i32)
                      n200 = local read "Adapted_XNum"() -> (w705:i32)
                      n201 = property on="Pressure Slope Map" class="IntGraph (strict)"("XScale.Maximum"=w705, "YScale.Maximum"=w704, "YScale.LooseFit"=w694, "XScale.LooseFit"=w694, "ZScale.LooseFit"=w694, "Smooth Update"=w692, "ZScale.ScaleFit"=w691) -> ()  [unwired: 2 in, 2 out]
                      n202 = node(w703, w699, "db_start_frame_timer" ("function name"), w702, w701) -> (w700:refnum<k35>, w698:errorcluster, w697:refnum<k38>)  [unwired: 2 in, 2 out]
                      n203 = property on="Topography" class="IntGraph (strict)"("XScale.Maximum"=w705, "YScale.Maximum"=w704, "YScale.LooseFit"=w694, "XScale.LooseFit"=w694, "ZScale.LooseFit"=w694, "Smooth Update"=w692, "ZScale.ScaleFit"=w691) -> ()  [unwired: 2 in, 2 out]
                    }
                    frame #1 {
                      w716 = 100000.0
                      w717 = -100000.0
                      # "TTH param structure:\n0, 1: X, Y piezo voltage\n2, 3: X, Y piezo idx\n4: Z piezo voltage\n5: baseline current\n6: circular buffer pointer idx\n(7-8106): Z voltage\n(8107-16206): current"
                      # "HTT param structure:\n0, 1: X, Y piezo voltage\n2, 3: X, Y piezo idx\n4: distance (piezo voltage) to the last point\n5: retract height, \nall negative cases won't trigger approach of z piezo\nif -20, keep z and move xy\nif -30, full retract for z and move xy"
                      n204 = local read "Adapted_XNum"() -> (w742:i32)
                      n205 = local read "Adapted_YNum"() -> (w741:i32)
                      n206 = Obtain Queue(name (unnamed)="data_array", element data type=dbl[] []) -> (queue out=w748:refnum<queue>)  [unwired: 3 in, 2 out]
                      n207 = New Data Value Reference(data value=FALSE) -> (data value reference=w749:refnum<data-value>)  [unwired: 1 in, 1 out]
                      n208 = Initialize Array(0.0, w742, w741) -> (w740:dbl[][])
                      n209 = flat-sequence {
                        tunnel: w749 -> [w1108]
                        tunnel: w748 -> [w1109]
                        tunnel: [w1109] -> w773
                        tunnel: [w1108] -> w771
                        tunnel: [w1107] -> w769
                        tunnel: [w1106] -> w766
                        tunnel: [w1101] -> w760
                        tunnel: [w1099] -> w759
                        tunnel: [w1094] -> w758
                        tunnel: [w1078] -> w757
                        tunnel: [w1091] -> w715
                        tunnel: [w1082] -> w714
                        tunnel: w713 -> [w1076]
                        tunnel: w712 -> [w1069]
                        tunnel: w711 -> [w1072]
                        tunnel: w710 -> [w1071]
                        tunnel: [w1073] -> w709
                        tunnel: [w1064] -> w708
                        tunnel: [w1163] -> w775
                        tunnel: [w1162] -> w774
                        tunnel: w773 -> [w1161]
                        tunnel: [w1161] -> w772
                        tunnel: w771 -> [w1154]
                        tunnel: [w1154] -> w770
                        tunnel: w769 -> [w1144]
                        tunnel: [w1156] -> w768
                        tunnel: [w1155] -> w767
                        tunnel: w766 -> [w1153]
                        tunnel: [w1153] -> w765
                        tunnel: [w1154] -> w764
                        tunnel: [w1152] -> w763
                        tunnel: [0] -> w762
                        tunnel: [w1150] -> w761
                        tunnel: w760 -> [w1149]
                        tunnel: w759 -> [w1148]
                        tunnel: w758 -> [w1147]
                        tunnel: w757 -> [w1145]
                        tunnel: [0] -> w751
                        tunnel: [w1145] -> w750
                        tunnel: w715 -> [w1143]
                        tunnel: w714 -> [w1142]
                        tunnel: w709 -> [_]
                        tunnel: w708 -> [_]
                        tunnel: w775 -> [w1189]
                        tunnel: w774 -> [w1188]
                        tunnel: w772 -> [w1187]
                        tunnel: w770 -> [w1186]
                        tunnel: w768 -> [w1185]
                        tunnel: w767 -> [w1184]
                        tunnel: w765 -> [w1183]
                        tunnel: w764 -> [w1182]
                        tunnel: w763 -> [w1181]
                        tunnel: w762 -> [w1180]
                        tunnel: w761 -> [w1179]
                        tunnel: [w1178] -> w756
                        tunnel: [w1177] -> w755
                        tunnel: [w1176] -> w754
                        tunnel: [w1175] -> w753
                        tunnel: w751 -> [w1174]
                        tunnel: w750 -> [w1173]
                        tunnel: [w1172] -> w733
                        tunnel: [w1171] -> w722
                        tunnel: [w1355] -> w732
                        tunnel: [w1354] -> w730
                        tunnel: [w1353] -> w728
                        tunnel: [w1351] -> w726
                        tunnel: w733 -> [w1350]
                        tunnel: w753 -> [w1352]
                        tunnel: w754 -> [w1353]
                        tunnel: w755 -> [w1354]
                        tunnel: w756 -> [w1355]
                        tunnel: w722 -> [w1349]
                        tunnel: [w1349] -> w720
                        tunnel: w732 -> [w1369]
                        tunnel: [w1369] -> w731
                        tunnel: w730 -> [w1368]
                        tunnel: [w1368] -> w729
                        tunnel: w728 -> [w1367]
                        tunnel: [w1367] -> w727
                        tunnel: w726 -> [w1366]
                        tunnel: [w1366] -> w725
                        tunnel: [w1364] -> w721
                        tunnel: w720 -> [w1364]
                        tunnel: w731 -> [w1371]
                        tunnel: w729 -> [w1370]
                        tunnel: w727 -> [w1375]
                        tunnel: w725 -> [w1374]
                        tunnel: [w1374] -> w752
                        tunnel: [w1373] -> w735
                        tunnel: w721 -> [w1372]
                        tunnel: [w1372] -> w719
                        frame #0 {
                          n210 = local read "ScanMode"() -> (w1077:i32)
                          n211 = local read "FrameNum"() -> (w1068:u32)
                          n212 = Equal?(x=w1077, y=3) -> (x = y?=w1057:bool)
                          n213 = Decrement(x=w1068) -> (x-1=w1067:u32)
                          n214 = Decrement(x=w1071) -> (x-1=w1070:i32)
                          n215 = local read "Adapted_XNum"() -> (w1093:i32)
                          n216 = local read "Adapted_YNum"() -> (w1092:i32)
                          n217 = Equal?(x=w1072, y=w1070) -> (x = y?=w1065:bool)
                          n218 = Equal To 0?(x=w1072) -> (x = 0?=w1075:bool)
                          n219 = Equal To 0?(x=w1069) -> (x = 0?=w1074:bool)
                          n220 = case shown="3" w1077 {
                            tunnel: [w1110 w1119 w1127 w1138] -> w1106
                            tunnel: w1076 -> [_ _ _ _]
                            frame 0, Default {
                              n221 = local read "Adapted_XNum"() -> (w1117:i32)
                              n222 = local read "Adapted_YNum"() -> (w1116:i32)
                              n223 = local read "Adapted_YOffset um"() -> (w1113:dbl)
                              n224 = local read "Adapted_XOffset um"() -> (w1112:dbl)
                              n225 = local read "Retract (flat) um"() -> (w1111:dbl)
                              n226 = local read "XStepSize um"() -> (w1115:dbl)
                              n227 = local read "YStepSize um"() -> (w1114:dbl)
                              n228 = call "xy_raster_scan.vi"("Retract um"=w1111, "YOffset um"=w1113, "XOffset um"=w1112, "YStepSize um"=w1114, "XStepSize um"=w1115, "YNum"=w1116, "XNum"=w1117) -> ("Converted_HTT_Params"=w1110:fxp<+/-,48,16>[])  [unwired: 4 in]
                            }
                            frame 1 {
                              n229 = local read "Adapted_XOffset um"() -> (w1123:dbl)
                              n230 = local read "Adapted_YOffset um"() -> (w1120:dbl)
                              n231 = local read "Retract (edge) um"() -> (w1118:dbl)
                              n232 = local read "Adapted_XNum"() -> (w1125:i32)
                              n233 = local read "Adapted_YNum"() -> (w1124:i32)
                              n234 = local read "XStepSize um"() -> (w1122:dbl)
                              n235 = local read "YStepSize um"() -> (w1121:dbl)
                              n236 = call "xy_raster_scan.vi"("Retract um"=w1118, "YOffset um"=w1120, "XOffset um"=w1123, "YStepSize um"=w1121, "XStepSize um"=w1122, "YNum"=w1124, "XNum"=w1125) -> ("Converted_HTT_Params"=w1119:fxp<+/-,48,16>[])  [unwired: 4 in]
                            }
                            frame 2 {
                              n237 = local read "Adapted_XOffset um"() -> (w1131:dbl)
                              n238 = local read "Adapted_YOffset um"() -> (w1128:dbl)
                              n239 = local read "Retract (edge) um"() -> (w1126:dbl)
                              n240 = local read "Adapted_XNum"() -> (w1133:i32)
                              n241 = local read "Adapted_YNum"() -> (w1132:i32)
                              n242 = local read "XStepSize um"() -> (w1130:dbl)
                              n243 = local read "YStepSize um"() -> (w1129:dbl)
                              n244 = call "xy_raster_scan.vi"("Retract um"=w1126, "YOffset um"=w1128, "XOffset um"=w1131, "YStepSize um"=w1129, "XStepSize um"=w1130, "YNum"=w1132, "XNum"=w1133) -> ("Converted_HTT_Params"=w1127:fxp<+/-,48,16>[])  [unwired: 4 in]
                            }
                            frame 3 {
                              w1137 = 0.0 ("XStepSize um")
                              w1134 = 1 ("YNum")
                              w1135 = 400 ("XNum")
                              n245 = local read "XOffset um"() -> (w1139:dbl)
                              n246 = local read "YOffset um"() -> (w1140:dbl)
                              n247 = local write "Adapted_XNum"(w1135) -> ()
                              n248 = local write "Adapted_YNum"(w1134) -> ()
                              n249 = call "xy_raster_scan.vi"("Retract um"=2.0, "YOffset um"=w1140, "XOffset um"=w1139, "YStepSize um"=w1137, "XStepSize um"=w1137, "YNum"=w1134, "XNum"=w1135) -> ("Converted_HTT_Params"=w1138:fxp<+/-,48,16>[])  [unwired: 4 in]
                            }
                          }
                          n250 = And(x=w1075, y=w1074) -> (x .and. y?=w1073:bool)
                          n251 = Equal?(x=w1069, y=w1067) -> (x = y?=w1066:bool)
                          n252 = Multiply(x=w1093, y=w1092) -> (x*y=w1080:i32)
                          n253 = local read "NF_AppRate um/s"() -> (w1060:dbl)
                          n254 = local read "FF_AppRate um/s"() -> (w1056:dbl)
                          n255 = local read "RetRate um/s"() -> (w1063:dbl)
                          n256 = local read "NF_Threshold %"() -> (w1086:dbl)
                          n257 = local read "FF_Threshold %"() -> (w1090:dbl)
                          n258 = Select(t=400, s=w1057, f=w1080) -> (s? t:f=w1078:i32)
                          n259 = And(x=w1066, y=w1065) -> (x .and. y?=w1064:bool)
                          n260 = Divide(x=25.0, y=0.032768) -> (x/y=w1095:dbl)
                          n261 = Select(t=15.0, s=w1057, f=w1063) -> (s? t:f=w1061:dbl)
                          n262 = Select(t=3.0, s=w1057, f=w1060) -> (s? t:f=w1058:dbl)
                          n263 = Select(t=5.0, s=w1057, f=w1056) -> (s? t:f=w1054:dbl)
                          n264 = Divide(x=w1090, y=100.0) -> (x/y=w1089:dbl)
                          n265 = Divide(x=w1086, y=100.0) -> (x/y=w1085:dbl)
                          n266 = Divide(x=w1095, y=w1054) -> (x/y=w1103:dbl)
                          n267 = Divide(x=w1095, y=w1058) -> (x/y=w1096:dbl)
                          n268 = Divide(x=w1095, y=w1061) -> (x/y=w1098:dbl)
                          n269 = Select(t=2, s=w1057, f=1) -> (s? t:f=w1082:i32)
                          n270 = Round To Nearest(number=w1103) -> (nearest integer value=w1102:dbl)
                          n271 = To Fixed-Point(number=w1089) -> (fixed-point=w1107:fxp<+/-,48,16>)  [unwired: 1 in]
                          n272 = To Fixed-Point(number=w1085) -> (fixed-point=w1091:fxp<+/-,48,16>)  [unwired: 1 in]
                          n273 = Round To Nearest(number=w1096) -> (nearest integer value=w1100:dbl)
                          n274 = Round To Nearest(number=w1098) -> (nearest integer value=w1097:dbl)
                          n275 = To Long Integer(number=w1100) -> (32bit integer=w1099:i32)
                          n276 = To Long Integer(number=w1097) -> (32bit integer=w1094:i32)
                          n277 = To Long Integer(number=w1102) -> (32bit integer=w1101:i32)
                        }
                        frame #1 {
                          w1141 = TRUE ("InitScan")
                          n278 = xnode "Open FPGA VI Reference"("resource name"=tag "RIO0") -> ("FPGA VI Reference Out"=w1160:refnum<k20>, "error out"=w1159:errorcluster)  [unwired: 1 in]
                          n279 = xnode "Read/Write Control"("FPGA VI Reference In"=w1160, "error in"=w1159, "Recording Threshold"=w1144, "Halting Threshold"=w1143, "AppRate_FF us"=w1149, "AppRate_NF us"=w1148, "RetRate us"=w1147, "TotalPoints"=w1145, "DelayPoints"=w1142, "InitScan"=w1141, "LastScan"=w1141) -> ("FPGA VI Reference Out"=w1169:refnum<k20>, "error out"=w1168:errorcluster)
                          n280 = xnode "Invoke Method"("FPGA VI Reference In"=w1160, "error in"=w1159, "Data"=fxp<+/-,48,16>[] [], "Timeout (ms)"=0) -> ("FPGA VI Reference Out"=w1156:refnum<k20>, "error out"=w1155:errorcluster, "Empty Elements Remaining"=w1150:u32)
                          n281 = Scale By Power Of 2(n=u32 18 ("Requested Depth"), x=u32 1 ("Requested Depth")) -> (x*2^n=w1165:u32)
                          n282 = xnode "Invoke Method"("FPGA VI Reference In"=w1169, "error in"=w1168, "Requested Depth"=w1165) -> ("FPGA VI Reference Out"=w1163:refnum<k20>, "error out"=w1162:errorcluster, "Actual Depth"=→"FPGA_Host_Buf_Depth":u32)
                          n283 = Array Size(array=w1153) -> (size(s)=w1152:i32)
                        }
                        frame #2 {
                          n284 = while {
                            tunnel: w1185 -> [w1207]
                            tunnel: w1184 -> [w1206]
                            tunnel: w1183 -> [w1203]
                            tunnel: w1182 -> [w1202]
                            tunnel: w1181 -> [w1201]
                            shift-right: [w1194] -> _
                            shift-left: w1180 -> [w1200]
                            tunnel: w1179 -> [w1199]
                            stop <- w1190 stop-if-true
                            n285 = flat-sequence {
                              tunnel: w1207 -> [w1231]
                              tunnel: w1206 -> [w1230]
                              tunnel: [w1225] -> w1205
                              tunnel: [w1224] -> w1204
                              tunnel: w1203 -> [w1213]
                              tunnel: w1202 -> [w1223]
                              tunnel: w1201 -> [w1222]
                              tunnel: w1200 -> [w1217]
                              tunnel: w1199 -> [w1221]
                              tunnel: [w1217] -> w1198
                              tunnel: [w1214] -> w1197
                              tunnel: [w1213] -> w1196
                              tunnel: [w1209] -> w1193
                              tunnel: [w1208] -> w1192
                              tunnel: w1205 -> [w1240]
                              tunnel: w1204 -> [w1239]
                              tunnel: w1198 -> [w1238]
                              tunnel: w1197 -> [w1237]
                              tunnel: w1196 -> [w1236]
                              tunnel: [w1235] -> w1195
                              tunnel: w1193 -> [w1234]
                              tunnel: w1192 -> [w1233]
                              tunnel: [w1233] -> w1191
                              tunnel: w1195 -> [w1251]
                              tunnel: [w1251] -> w1194
                              tunnel: w1191 -> [w1250]
                              tunnel: [w1250] -> w1190
                              frame #0 {
                                w1215 = u32 128 ("y")
                                n286 = in-place {
                                in-place-border: [w1232] -> w1211
                                n287 = in-place-dvr #1(w1223) -> (w1232:bool)  [unwired: 1 out]
                                n288 = in-place-dvr #1(w1232) -> ()  [unwired: 2 out]
                                }
                                n289 = xnode "Invoke Method"("FPGA VI Reference In"=w1231, "error in"=w1230, "Data"=fxp<+/-,48,16>[] [], "Timeout (ms)"=0) -> ("FPGA VI Reference Out"=w1227:refnum<k20>, "error out"=w1226:errorcluster, "Empty Elements Remaining"=w1220:u32)
                                n290 = Subtract(x=w1222, y=w1217) -> (x-y=w1216:u32)
                                n291 = Subtract(x=w1221, y=w1220) -> (x-y=w1219:u32)
                                n292 = Less Or Equal?(x=w1219, y=w1215) -> (x <= y?=w1218:bool)
                                n293 = Less Or Equal?(x=w1216, y=w1215) -> (x <= y?=w1210:bool)
                                n294 = Or(x=w1218, y=w1210) -> (x .or. y?=w1209:bool)
                                n295 = xnode "Read/Write Control"("FPGA VI Reference In"=w1227, "error in"=w1226) -> ("FPGA VI Reference Out"=w1225:refnum<k20>, "error out"=w1224:errorcluster, "TargetDone?"=w1212:bool)
                                n296 = Select(t=w1216, s=w1210, f=w1215) -> (s? t:f=w1214:u32)
                                n297 = Compound Arithmetic op=OR(w1212, w1210, w1211) -> (w1208:bool)
                              }
                              frame #1 {
                                n298 = case shown="True" w1234 {
                                tunnel: w1240 -> [_ w1249]
                                tunnel: w1239 -> [_ w1248]
                                tunnel: w1238 -> [w1241 w1244]
                                tunnel: w1237 -> [_ w1243]
                                tunnel: w1236 -> [_ w1245]
                                tunnel: [w1241 w1246] -> w1235
                                frame False {
                                }
                                frame True {
                                n299 = Array Subset(array=w1245, index=w1244, length=w1243) -> (w1242:fxp<+/-,48,16>[])
                                n300 = Add(x=w1243, y=w1244) -> (x+y=w1246:u32)
                                "HTT_Buffer_Write" <- w1246
                                n301 = xnode "Invoke Method"("FPGA VI Reference In"=w1249, "error in"=w1248, "Data"=w1242, "Timeout (ms)"=10000) -> ()  [unwired: 3 out]
                                }
                                }
                              }
                              frame #2 {
                                n302 = Wait (ms)(milliseconds to wait=u32 100) -> ()  [unwired: 1 out]
                              }
                            }
                          }
                          n303 = while {
                            tunnel: w1189 -> [w1282]
                            tunnel: w1188 -> [w1281]
                            tunnel: w1187 -> [w1278]
                            tunnel: w1186 -> [w1277]
                            tunnel: [w1270] -> w1178
                            tunnel: [w1269] -> w1177
                            tunnel: [w1267] -> w1176
                            tunnel: [w1265] -> w1175
                            shift-right: [w1261] -> _
                            shift-left: w1174 -> [w1264]
                            tunnel: w1173 -> [w1257]
                            tunnel: [w1254] -> w1172
                            tunnel: [w1253] -> w1171
                            stop <- w1258 stop-if-true
                            n304 = flat-sequence {
                              tunnel: w1282 -> [w1301]
                              tunnel: w1281 -> [w1300]
                              tunnel: [w1295] -> w1280
                              tunnel: [w1294] -> w1279
                              tunnel: w1278 -> [w1290]
                              tunnel: w1277 -> [w1288]
                              tunnel: [w1290] -> w1276
                              tunnel: [w1289] -> w1275
                              tunnel: [w1287] -> w1274
                              tunnel: [w1286] -> w1271
                              tunnel: w1264 -> [w1285]
                              tunnel: [w1285] -> w1263
                              tunnel: [w1283] -> w1260
                              tunnel: w1257 -> [w1284]
                              tunnel: [w1284] -> w1256
                              tunnel: w1280 -> [w1315]
                              tunnel: w1279 -> [w1314]
                              tunnel: w1276 -> [w1313]
                              tunnel: w1275 -> [w1312]
                              tunnel: w1274 -> [w1311]
                              tunnel: [w1310] -> w1273
                              tunnel: [w1309] -> w1272
                              tunnel: w1271 -> [w1308]
                              tunnel: [w1308] -> w1268
                              tunnel: [w1307] -> w1266
                              tunnel: w1263 -> [w1306]
                              tunnel: [w1305] -> w1262
                              tunnel: w1260 -> [w1304]
                              tunnel: [w1304] -> w1259
                              tunnel: w1256 -> [w1303]
                              tunnel: [w1303] -> w1255
                              tunnel: w1273 -> [w1347]
                              tunnel: w1272 -> [w1346]
                              tunnel: [w1347] -> w1270
                              tunnel: [w1346] -> w1269
                              tunnel: [w1345] -> w1267
                              tunnel: w1268 -> [w1345]
                              tunnel: w1266 -> [w1344]
                              tunnel: [w1344] -> w1265
                              tunnel: w1262 -> [w1342]
                              tunnel: [w1342] -> w1261
                              tunnel: w1259 -> [w1340]
                              tunnel: [w1343] -> w1258
                              tunnel: w1255 -> [w1341]
                              tunnel: [w1340] -> w1254
                              tunnel: [w1339] -> w1253
                              frame #0 {
                                w1293 = 16384
                                w1297 = u32 0 ("Number of Elements")
                                n305 = in-place {
                                in-place-border: [w1302] -> w1283
                                n306 = in-place-dvr #2(w1288) -> (w1302:bool)  [unwired: 1 out]
                                n307 = in-place-dvr #2(w1302) -> (w1286:refnum<data-value>)  [unwired: 1 out]
                                }
                                n308 = xnode "Read/Write Control"("FPGA VI Reference In"=w1301, "error in"=w1300, "stop"=w1283) -> ("FPGA VI Reference Out"=w1299:refnum<k20>, "error out"=w1298:errorcluster)
                                n309 = xnode "Invoke Method"("FPGA VI Reference In"=w1299, "error in"=w1298, "Number of Elements"=w1297, "Timeout (ms)"=w1297) -> ("FPGA VI Reference Out"=w1295:refnum<k20>, "error out"=w1294:errorcluster, "Elements Remaining"=w1296:u32)  [unwired: 1 out]
                                n310 = Quotient & Remainder(x=w1296, y=w1293) -> (floor(x/y)=w1292:u32)  [unwired: 1 out]
                                n311 = Multiply(x=w1293, y=w1292) -> (x*y=w1287:u32)
                                n312 = Greater Than 0?(x=w1292) -> (x > 0?=w1291:bool)
                                n313 = Compound Arithmetic op=AND(w1291, invert w1283) -> (w1289:bool)
                              }
                              frame #1 {
                                n314 = case shown="True" w1312 {
                                tunnel: w1315 -> [w1319 w1335]
                                tunnel: w1314 -> [w1318 w1334]
                                tunnel: w1313 -> [w1317 w1328]
                                tunnel: w1311 -> [_ w1330]
                                tunnel: [w1319 w1332] -> w1310
                                tunnel: [w1318 w1331] -> w1309
                                tunnel: [w1317 w1323] -> w1307
                                tunnel: w1306 -> [w1316 w1322]
                                tunnel: [w1316 w1320] -> w1305
                                frame False {
                                }
                                frame True {
                                w1325 = 16384
                                n315 = xnode "Invoke Method"("FPGA VI Reference In"=w1335, "error in"=w1334, "Number of Elements"=w1330, "Timeout (ms)"=10000) -> ("FPGA VI Reference Out"=w1332:refnum<k20>, "error out"=w1331:errorcluster, "Data"=w1329:fxp<+/-,48,16>[])  [unwired: 1 out]
                                n316 = To Double Precision Float(number=w1329) -> (double precision float=w1326:dbl[])
                                n317 = Array Size(array=w1326) -> (size(s)=w1327:i32)
                                n318 = Quotient & Remainder(x=w1327, y=w1325) -> (floor(x/y)=w1321:i32)  [unwired: 1 out]
                                n319 = Add(x=w1322, y=w1321) -> (x+y=w1320:i32)
                                n320 = Reshape Array(w1326, w1321, w1325) -> (w1324:dbl[][])
                                n321 = for {
                                N: w1321 -> [_]
                                tunnel: w1328 -> [w1338]
                                tunnel: w1324 -> [w1337] mode=indexing
                                tunnel: [w1336] -> w1323
                                n322 = Enqueue Element(queue=w1338, element=w1337) -> (queue out=w1336:refnum<queue>)  [unwired: 2 in, 2 out]
                                }
                                }
                                }
                              }
                              frame #2 {
                                n323 = Greater Or Equal?(x=w1342, y=w1341) -> (x >= y?=w1339:bool)
                                n324 = Wait (ms)(milliseconds to wait=u32 20) -> ()  [unwired: 1 out]
                                n325 = Or(x=w1339, y=w1340) -> (x .or. y?=w1343:bool)
                                "Scanned Points" <- w1342
                              }
                            }
                          }
                        }
                        frame #3 {
                          n326 = case shown="False" w1350 {
                            tunnel: w1352 -> [w1357 w1363]
                            tunnel: [w1356 w1363] -> w1351
                            frame False {
                              n327 = while {
                                tunnel: w1357 -> [w1362]
                                tunnel: [w1361] -> w1356
                                stop <- w1359 stop-if-true
                                n328 = Get Queue Status(queue=w1362) -> (queue out=w1361:refnum<queue>, # elements in queue=w1360:i32)  [unwired: 2 in, 6 out]
                                n329 = Less Or Equal To 0?(x=w1360) -> (x <= 0?=w1359:bool)
                                n330 = Wait (ms)(milliseconds to wait=u32 100) -> ()  [unwired: 1 out]
                              }
                            }
                            frame True {
                            }
                          }
                        }
                        frame #4 {
                          n331 = Wait (ms)(milliseconds to wait=u32 500) -> ()  [unwired: 1 out]
                        }
                        frame #5 {
                          n332 = in-place {
                            n333 = in-place-dvr #3(w1375) -> ()  [unwired: 2 out]
                            n334 = in-place-dvr #3(TRUE ("data value")) -> (w1373:refnum<data-value>)  [unwired: 1 out]
                          }
                          n335 = xnode "Close FPGA VI Reference"("FPGA VI Reference In"=w1371, "error in"=w1370) -> ()  [unwired: 1 out]
                        }
                      }
                      n336 = flat-sequence {
                        tunnel: w749 -> [w801]
                        tunnel: w748 -> [w800]
                        tunnel: w747 -> [w799]
                        tunnel: w746 -> [w798]
                        tunnel: w745 -> [w797]
                        tunnel: w744 -> [w796]
                        tunnel: [w795] -> w739
                        tunnel: [w794] -> w738
                        tunnel: [w793] -> w737
                        tunnel: [w792] -> w736
                        tunnel: w712 -> [w791]
                        tunnel: w740 -> [w790]
                        tunnel: w740 -> [w789]
                        tunnel: w717 -> [w788]
                        tunnel: w716 -> [w787]
                        tunnel: w717 -> [w786]
                        tunnel: w716 -> [w785]
                        tunnel: [w784] -> w734
                        tunnel: w724 -> [w783]
                        tunnel: [w782] -> w723
                        tunnel: [w781] -> w718
                        tunnel: w711 -> [w780]
                        tunnel: [w779] -> w707
                        frame #0 {
                          n337 = while {
                            tunnel: w801 -> [w864]
                            tunnel: w800 -> [w863]
                            tunnel: w799 -> [w862]
                            tunnel: w798 -> [w861]
                            tunnel: w797 -> [w860]
                            tunnel: w796 -> [w856]
                            tunnel: [w850] -> w795
                            tunnel: [w849] -> w794
                            tunnel: [w848] -> w793
                            tunnel: [w847] -> w792
                            tunnel: w791 -> [w843]
                            shift-right: [w833] -> _
                            shift-left: w790 -> [w841]
                            shift-right: [w831] -> _
                            shift-left: w789 -> [w836]
                            shift-right: [w821] -> _
                            shift-left: w788 -> [w830]
                            shift-right: [w819] -> _
                            shift-left: w787 -> [w829]
                            shift-right: [w817] -> _
                            shift-left: w786 -> [w826]
                            shift-right: [w815] -> _
                            shift-left: w785 -> [w825]
                            tunnel: [w812] -> w784
                            tunnel: w783 -> [w811]
                            tunnel: [w808] -> w782
                            tunnel: [w806] -> w781
                            tunnel: w780 -> [w805]
                            tunnel: [w802] -> w779
                            stop <- w838 stop-if-true
                            n338 = flat-sequence {
                              tunnel: w864 -> [w887]
                              tunnel: w863 -> [w882]
                              tunnel: w862 -> [w886]
                              tunnel: w861 -> [w885]
                              tunnel: w860 -> [w884]
                              tunnel: [w886] -> w859
                              tunnel: [w885] -> w858
                              tunnel: [w884] -> w857
                              tunnel: w856 -> [w883]
                              tunnel: [w883] -> w855
                              tunnel: [w881] -> w846
                              tunnel: [w880] -> w845
                              tunnel: [w879] -> w844
                              tunnel: w843 -> [w878]
                              tunnel: [w878] -> w842
                              tunnel: w841 -> [w876]
                              tunnel: [w877] -> w840
                              tunnel: [w876] -> w837
                              tunnel: w836 -> [w875]
                              tunnel: [w875] -> w835
                              tunnel: w830 -> [w874]
                              tunnel: w829 -> [w873]
                              tunnel: [w874] -> w828
                              tunnel: [w873] -> w827
                              tunnel: w826 -> [w872]
                              tunnel: w825 -> [w871]
                              tunnel: [w872] -> w824
                              tunnel: [w871] -> w823
                              tunnel: [w870] -> w814
                              tunnel: w811 -> [w869]
                              tunnel: [w866] -> w810
                              tunnel: w805 -> [w865]
                              tunnel: [w865] -> w804
                              tunnel: w859 -> [w920]
                              tunnel: w858 -> [w919]
                              tunnel: w857 -> [w918]
                              tunnel: w855 -> [w917]
                              tunnel: [w916] -> w854
                              tunnel: [w915] -> w853
                              tunnel: [w914] -> w852
                              tunnel: [w913] -> w851
                              tunnel: w846 -> [w912]
                              tunnel: w845 -> [w911]
                              tunnel: w844 -> [w910]
                              tunnel: w842 -> [w909]
                              tunnel: w840 -> [w908]
                              tunnel: [w908] -> w839
                              tunnel: w837 -> [w907]
                              tunnel: w835 -> [w906]
                              tunnel: [w905] -> w834
                              tunnel: [w904] -> w832
                              tunnel: w828 -> [w903]
                              tunnel: w827 -> [w902]
                              tunnel: w824 -> [w901]
                              tunnel: w823 -> [w900]
                              tunnel: [w899] -> w822
                              tunnel: [w898] -> w820
                              tunnel: [w897] -> w818
                              tunnel: [w896] -> w816
                              tunnel: w814 -> [w895]
                              tunnel: [w895] -> w813
                              tunnel: w810 -> [w894]
                              tunnel: [w894] -> w809
                              tunnel: [w893] -> w807
                              tunnel: w804 -> [w892]
                              tunnel: [w891] -> w803
                              tunnel: w854 -> [w1051]
                              tunnel: w853 -> [w1050]
                              tunnel: w852 -> [w1049]
                              tunnel: w851 -> [w1052]
                              tunnel: [w1052] -> w850
                              tunnel: [w1051] -> w849
                              tunnel: [w1050] -> w848
                              tunnel: [w1049] -> w847
                              tunnel: [w1048] -> w838
                              tunnel: w839 -> [w1048]
                              tunnel: w834 -> [w1047]
                              tunnel: [w1047] -> w833
                              tunnel: w832 -> [w1046]
                              tunnel: [w1046] -> w831
                              tunnel: w822 -> [w1045]
                              tunnel: [w1045] -> w821
                              tunnel: w820 -> [w1044]
                              tunnel: [w1044] -> w819
                              tunnel: w818 -> [w1043]
                              tunnel: [w1043] -> w817
                              tunnel: w816 -> [w1042]
                              tunnel: [w1042] -> w815
                              tunnel: w813 -> [w1041]
                              tunnel: [w1041] -> w812
                              tunnel: w809 -> [w1040]
                              tunnel: [w1040] -> w808
                              tunnel: w807 -> [w1039]
                              tunnel: [w1039] -> w806
                              tunnel: w803 -> [w1038]
                              tunnel: [w1038] -> w802
                              frame #0 {
                                # "topography max min"
                                # "pressure slope map"
                                # "topography"
                                n339 = Get Queue Status(queue=w869) -> (queue out=w866:refnum<queue>, # elements in queue=w868:i32)  [unwired: 2 in, 6 out]
                                n340 = Greater Than 0?(x=w868) -> (x > 0?=w867:bool)
                                n341 = Get Queue Status(queue=w882) -> (queue out=w880:refnum<queue>, # elements in queue=w879:i32)  [unwired: 2 in, 6 out]
                                n342 = in-place {
                                in-place-border: w867 -> [w888]
                                in-place-border: [w889] -> w877
                                in-place-border: [w888] -> w870
                                n343 = in-place-dvr #4(w887) -> (w890:bool)  [unwired: 1 out]
                                n344 = Or(x=w890, y=w888) -> (x .or. y?=w889:bool)
                                n345 = in-place-dvr #4(w889) -> ()  [unwired: 2 out]
                                }
                                n346 = Greater Than 0?(x=w879) -> (x > 0?=w881:bool)
                              }
                              frame #1 {
                                n347 = case shown="True" w912 {
                                tunnel: w920 -> [w931 w961]
                                tunnel: w919 -> [w930 w960]
                                tunnel: w918 -> [w929 w959]
                                tunnel: w917 -> [w932 w955]
                                tunnel: [w931 w958] -> w916
                                tunnel: [w930 w957] -> w915
                                tunnel: [w929 w956] -> w914
                                tunnel: [w932 w954] -> w913
                                tunnel: w911 -> [_ w952]
                                tunnel: w910 -> [_ w953]
                                tunnel: w909 -> [w922 w951]
                                tunnel: w907 -> [w928 w950]
                                tunnel: w906 -> [w927 w949]
                                tunnel: [w928 w936] -> w905
                                tunnel: [w927 w935] -> w904
                                tunnel: w903 -> [w926 w945]
                                tunnel: w902 -> [w925 w944]
                                tunnel: w901 -> [w924 w943]
                                tunnel: w900 -> [w923 w942]
                                tunnel: [w926 w941] -> w899
                                tunnel: [w925 w940] -> w898
                                tunnel: [w924 w939] -> w897
                                tunnel: [w923 w938] -> w896
                                tunnel: [w922 w937] -> w893
                                tunnel: w892 -> [w921 w934]
                                tunnel: [w921 w933] -> w891
                                frame False {
                                }
                                frame True {
                                n348 = for {
                                N: w953 -> [_]
                                tunnel: w955 -> [w1023]
                                tunnel: [w1023] -> w954
                                tunnel: w961 -> [w1030]
                                tunnel: [w1026] -> w958
                                tunnel: w960 -> [w1028]
                                tunnel: [w1025] -> w957
                                tunnel: w959 -> [w1027]
                                tunnel: [w1024] -> w956
                                tunnel: w952 -> [w1022]
                                tunnel: w951 -> [w963]
                                shift-right: [w988] -> w936
                                shift-left: w950 -> [w989]
                                shift-right: [w986] -> w935
                                shift-left: w949 -> [w987]
                                tunnel: [w971] -> w948
                                tunnel: [w972] -> w947
                                shift-right: [w984] -> w941
                                shift-left: w945 -> [w985]
                                shift-right: [w982] -> w940
                                shift-left: w944 -> [w983]
                                shift-right: [w978] -> w939
                                shift-left: w943 -> [w981]
                                shift-right: [w977] -> w938
                                shift-left: w942 -> [w980]
                                tunnel: [w976] -> w937
                                tunnel: w934 -> [w962]
                                tunnel: [w962] -> w933
                                w991 = T3 0 items=["Least Square", "Least Absolute Residual", "Bisquare"] ("method")
                                n349 = Dequeue Element(queue=w1022) -> (element=w1013:dbl[])  [unwired: 2 in, 3 out]
                                n350 = Array Subset(array=w1013, index=7, length=8100 ("index")) -> (w1006:dbl[])
                                n351 = Array Subset(array=w1013, index=8107, length=8100 ("index")) -> (w1007:dbl[])
                                n352 = Index Array(array=w1013, index #1=0 ("index"), index #2=1 ("index"), index #3=2 ("index"), index #4=3 ("index"), index #5=4 ("index"), index #6=5 ("index"), index #7=6 ("index")) -> (element #1=w1004:dbl, element #2=w1002:dbl, element #3=w1001:dbl, element #4=w999:dbl, element #5=w997:dbl, element #6=w969:dbl, element #7=w973:dbl)
                                n353 = To Long Integer(number=w973) -> (32bit integer=w970:i32)
                                n354 = Search 1D Array(1D array=w1006, element=-100.0) -> (index of element=w1005:i32)  [unwired: 1 in]
                                n355 = Equal?(x=w1005, y=-1) -> (x = y?=w1008:bool)
                                n356 = To Long Integer(number=w1001) -> (32bit integer=w966:i32)
                                n357 = To Long Integer(number=w999) -> (32bit integer=w967:i32)
                                n358 = case shown="False" w1008 {
                                tunnel: w1007 -> [w1034 w1036]
                                tunnel: w1006 -> [w1035 w1037]
                                tunnel: w1005 -> [w1031 _]
                                tunnel: [w1033 w1037] -> w992
                                tunnel: [w1032 w1036] -> w972
                                frame False {
                                n359 = Split 1D Array(array=w1035, index=w1031) -> (first subarray=w1033:dbl[])  [unwired: 1 out]
                                n360 = Split 1D Array(array=w1034, index=w1031) -> (first subarray=w1032:dbl[])  [unwired: 1 out]
                                }
                                frame True {
                                }
                                }
                                n361 = Multiply(x=w1004, y=10.0) -> (x*y=w964:dbl)
                                n362 = Multiply(x=w1002, y=10.0) -> (x*y=w965:dbl)
                                n363 = Multiply(x=w997, y=2.5) -> (x*y=w996:dbl)
                                n364 = Subtract(x=25.0, y=w996) -> (x-y=w968:dbl)
                                n365 = Multiply(x=w992, y=2.5) -> (x*y=w990:dbl[])
                                n366 = Array Size(array=w972) -> (size(s)=→"Signal Size":i32)
                                n367 = Subtract(x=25.0, y=w990) -> (x-y=w971:dbl[])
                                n368 = call <vilib>:"Linear Fit.vi"("Y"=w972, "X"=w971, "method"=w991) -> ("slope"=w979:dbl)  [unwired: 8 in, 4 out]
                                n369 = node(w1030, w1023, "db_insert_data" ("function name"), w1028, w1027, w962, w963, w964, w965, w966, w967, w968, w969, w970, w971, w972) -> (w1026:refnum<k35>, w1025:errorcluster, w1024:refnum<k38>, w976:i32)  [unwired: 12 in, 2 out]
                                n370 = Max & Min(x=w968, y=w985) -> (max(x,y)=w984:dbl)  [unwired: 1 out]
                                n371 = Max & Min(x=w983, y=w968) -> (min(x,y)=w982:dbl)  [unwired: 1 out]
                                n372 = Max & Min(x=w979, y=w981) -> (max(x,y)=w978:dbl)  [unwired: 1 out]
                                n373 = Max & Min(x=w980, y=w979) -> (min(x,y)=w977:dbl)  [unwired: 1 out]
                                n374 = Replace Array Subset(array=w987, new element=w979, index (row)=w966, index (col)=w967) -> (w986:dbl[][])
                                n375 = Replace Array Subset(array=w989, new element=w968, index (row)=w966, index (col)=w967) -> (w988:dbl[][])
                                }
                                n376 = Bundle(w948, w947) -> (→"IZCurve":cluster{dbl[], dbl[]})  [unwired: 1 in]
                                n377 = local write "Pressure Slope Map"(w935) -> ()
                                n378 = local write "Topography"(w936) -> ()
                                }
                                }
                              }
                              frame #2 {
                                n379 = Wait (ms)(milliseconds to wait=u32 50) -> ()  [unwired: 1 out]
                              }
                            }
                          }
                        }
                      }
                    }
                    frame #2 {
                      n380 = Delete Data Value Reference(data value reference=w1389) -> ()  [unwired: 1 in, 2 out]
                      n381 = Release Queue(queue=w1391) -> ()  [unwired: 2 in, 3 out]
                      n382 = node(w1388, w1386, "db_end_frame_timer" ("function name"), w1387, w1383, w1377, w1378, w1379) -> (w1385:refnum<k35>, w1384:errorcluster, w1382:refnum<k38>)  [unwired: 5 in, 2 out]
                    }
                  }
                }
              }
              frame #3 {
                n383 = local read "Adapted_XOffset um"() -> (w1393:dbl)
                n384 = local read "Adapted_YOffset um"() -> (w1392:dbl)
                n385 = local read "Adapted_YNum"() -> (w1396:i32)
                n386 = local read "Adapted_XNum"() -> (w1397:i32)
                n387 = local read "XStepSize um"() -> (w1395:dbl)
                n388 = local read "YStepSize um"() -> (w1394:dbl)
              }
            }
          }
        }
        frame #5 {
          n389 = local read "Retract (edge) um"() -> (w1414:dbl)
          n390 = local read "NF_AppRate um/s"() -> (w1416:dbl)
          n391 = local read "FF_AppRate um/s"() -> (w1415:dbl)
          n392 = node(w1428, w1422, "db_end_global_timer" ("function name"), w1427, w1426) -> (w1425:refnum<k35>, w1424:errorcluster, w1423:refnum<k38>)  [unwired: 2 in, 2 out]
          n393 = local read "Retract (flat) um"() -> (w1417:dbl)
          n394 = local read "FF_Threshold %"() -> (w1419:dbl)
          n395 = local read "NF_Threshold %"() -> (w1418:dbl)
          n396 = local read "Pressure kPa"() -> (w1412:dbl)
          n397 = local read "FrameNum"() -> (w1411:u32)
          n398 = local read "Notes"() -> (w1413:string)
          n399 = node(w1425, w1422, "db_insert_info" ("function name"), w1424, w1423, 0, w1409, w1408, w1407, w1406, w1405, w1404, w1419, w1418, w1417, w1414, w1415, w1416, w1410, w1411, w1412, w1413) -> (w1432:refnum<k35>, w1431:errorcluster, w1430:refnum<k38>)  [unwired: 19 in, 2 out]
          n400 = Close Python Session(session in=w1432, error in=w1431) -> ()  [unwired: 1 out]
          n401 = Close Reference(reference=w1430) -> ()  [unwired: 1 in, 1 out]
        }
        frame #6 {
          n402 = local write "Done?"(TRUE ("Done?")) -> ()
        }
      }
      n403 = while {
        tunnel: w30 -> [w41]
        stop <- w43 stop-if-true
        n404 = local read "Done?"() -> (w44:bool)
        n405 = Or(x="stop", y=w44) -> (x .or. y?=w43:bool)
        n406 = case shown="True" "stop" {
          tunnel: w41 -> [_ w46]
          tunnel: "stop" -> [_ w45]
          frame False {
          }
          frame True {
            n407 = Lossy Enqueue Element(queue=w46, element=w45) -> ()  [unwired: 1 in, 4 out]
          }
        }
        n408 = Wait (ms)(milliseconds to wait=u32 50) -> ()  [unwired: 1 out]
      }
    }
    frame #2 {
      n409 = Release Queue(queue=w1436) -> ()  [unwired: 2 in, 3 out]
    }
  }
